vi "Module - Page Setup.vi"(11 "Stop":bool) -> ()   [LabVIEW 2020]
uses:
  Control/Setup - Sequence Data v2.ctl
  Control/Setup - Single Sequence.ctl
  Control/Setup - State.ctl
  Control/Data to Execute.ctl
  Control/Transaction Info.ctl
  Control/Product Info.ctl
  Control/Acceptance Criteria Info.ctl
  Control/Execution Info.ctl
  Control/Results Info.ctl
  Control/State - FGV.ctl
  Control/State - eFGV.ctl
  Control/Section.ctl
  <vilib>/Utility/NIReport.llb/Report Type.ctl
  7311f70c-db24-4098-937e-a840d3f1464f.vi
  babc2730-5d00-47f3-8067-32ba08f41054.vi
  3b850bdc-189a-44ac-97c7-3d94fde3370d.vi
  472a6105-114d-4794-aef6-48c339f41fe4.vi
  b5994df8-9a62-4c2b-b0b7-1cda760cb50f.vi
  133289ce-597c-4077-9071-527faaeab83e.vi
  50162af0-f45e-4f35-a68f-88f28c3fa732.vi
  <vilib>/Utility/config.llb/Read Key (String).vi
  <vilib>/addons/_office/excel.llb/Excel Get Data ([str]).vi
  <vilib>/Comparison/Equal/Equal Functor/Equal Functor.lvclass
  <vilib>/Comparison/Less/Less Functor/Less Functor.lvclass
  <vilib>/Utility/NIReport.llb/NI_report.lvclass
  <vilib>/Utility/config.llb/NI_LVConfig.lvlib
  <vilib>/Utility/file.llb/Read Delimited Spreadsheet (string).vi
  <vilib>/Utility/NIReport.llb/NI_ReportGenerationCore.lvlib
  <vilib>/Utility/NIReport.llb/Excel/NI_Excel.lvclass
  <vilib>/addons/_office/NI_ReportGenerationToolkit.lvlib
panel:
  out "Label.Test System":string="Test System"
  out "Label.Working Pressure":string="Working Pressure"
  out "Label.Test Doc No":string="Test Doc. No./Ref."
  out "Label.Product Category":string="Product Category "
  out "Label.NCR No":string="NCR No."
  out "Label.Operation No":string="Operation No.*"
  out "Label.Material":string="Material*"
  out "Label.Customer":string="Customer"
  out "Label.Project":string="Project*"
  out "Label.RefOrderNo":string="Ref. Order No.*"
  out "Label.OrderNumber":string="Order Number*"
  out "Run No.":string="99"
  in  "Label.Sensor 3":string="Sensor" caption="Sensor"
  in  "Add Additional Ref Procedure":bool caption="Add Sensor"
  in  "Remove Additional Ref Procedure":bool caption="Remove Sensor"
  in  "Table.Procedure No./Ref.":i32(listbox)
  in  "Listbox.PSL":string(combo) caption="PSL"
  in  "Listbox.Rev.":string(combo) caption="Rev."
  in  "Listbox.Additional Procedures No./Ref.":string(combo) caption="Additional Procedures No./Ref."
  in  "Label.Production Order Details":string="Production Order Details" caption="Production Order Details"
  out "Indicator.Sub Operation":string caption="Sub Operation"
  out "Indicator.Confirmation No":u32 caption="Confirmation No"
  out "Indicator.Operation":string caption="Operation"
  out "Indicator.Sequence No":u16 caption="Sequence No"
  out "Indicator.Order Number":u32 caption="Order Number"
  in  "Desc.TestSystem":string="SUT1"
  in  "Desc.ProductCategory":string="Single Unit Test"
  out "1D Results":string[](array[string])
  in  "Label.Sensor 2":string="Sensor" caption="Sensor"
  in  "Enum.Pressure stabilize wait time":enum16{"seconds", "minutes"}(ring)
  in  "Pressure stabilize wait time":dbl=30.0 caption="Test Pressure Drop Rate every" min=0.0 max=100.0
  in  "Enum.Permitted Hold Pressure Drop":enum16{"%", "psi"}(ring)
  in  "Enum.Max Start Hold Pressure":enum16{"%", "psi"}(ring)
  in  "Permitted Hold Pressure Drop":dbl=3.0 caption="Permitted Holding Pressure Drop" min=0.0 max=100.0
  in  "Max Start Hold Pressure":dbl=3.0 caption="Maximum Start of Holding Pressure" min=0.0 max=100.0
  in  "Sales Order":string
  in  "Item No.":string
  in  "Customer":string
  in  "NCR No. 2":string caption="Operation No.*"
  in  "Load Excel":bool
  in  "template (empty)":path
  in  "Tab Control":enum32{"Test", "Misc."}(tab)
  in  "ComboBox.SelectTestSequence":string(combo) caption="Test Sequence"
  in  "Remove Multi test":bool caption="Remove Sensor"
  in  "Add Multi test":bool caption="Add Sensor"
  out "Setup-Sequence Data":T1={"Seq.Done"="\nSts.", "Label.RunSeq"="\nRun", "Label.TestSeq"="Test Seq.", "Label.SeqNo"="\nNo.", "Seq.No 5"="\nTest Requirement", "Seq.No 6"="\nVariance", "Seq.No 7"="Test\nProcedure", "Seq.No 8"="\nSect.", "Seq.No 9"="Test\nSystem", "Seq.No 10"="\nTest Media", "Seq.No 11"="Test Pressure ", "Seq.No 12"="\nCycle", "Seq.No 13"="Hold. time\n(hh:mm)", "Seq.No 14"="\nChart Scale", "Seq.No 15"="\nBD", "Seq.No 16"="Actuator\nPressure", "Seq.No 17"="Max. BD\nPressure", "Label.SelectSeq"="\nSel.", "Bool.SelectSeq"=TRUE, "Bool.RunSeq"=FALSE, "Bool.TestSeq"=TRUE, "Bool.SeqNo"=FALSE, "Label.TestGroup"="Test Grp.", "Bool.TestGroup"=FALSE, "Seq.MSHP"="MSHP\n(%)", "Seq.PHPD"="PHPD\n(%)", "Array"=[{"Seq.Select"=TRUE, "Seq.Status"=16777215, "Seq.Run"=FALSE, "Seq.TestSequence"="", "Seq.No"="", "Seq.TestReq"="", "Seq.TestProcedure"="", "Seq.Section"="", "Seq.TestPressure"="88,888", "Seq.TestGroup"="", "Seq.MSHP"=0.0, "Seq.PHPD"=0.0, "Seq.HoldingTime"="", "Seq.ChartScale"="", "Seq.ActuatorPressure"="", "Seq.MaxBDPressure"="", "Seq.BDIndicator"=FALSE, "Seq.TestMedia"="", "Seq.Variance"="AMV", "Seq.TestCycle"="", "Seq.TestSystem"=""}, {"Seq.Select"=TRUE, "Seq.Status"=16777215, "Seq.Run"=FALSE, "Seq.TestSequence"="", "Seq.No"="", "Seq.TestReq"="", "Seq.TestProcedure"="", "Seq.Section"="", "Seq.TestPressure"="", "Seq.TestGroup"="", "Seq.MSHP"=0.0, "Seq.PHPD"=0.0, "Seq.HoldingTime"="", "Seq.ChartScale"="", "Seq.ActuatorPressure"="", "Seq.MaxBDPressure"="", "Seq.BDIndicator"=FALSE, "Seq.TestMedia"="", "Seq.Variance"="AAV", "Seq.TestCycle"="", "Seq.TestSystem"=""}, {"Seq.Select"=TRUE, "Seq.Status"=16777215, "Seq.Run"=FALSE, "Seq.TestSequence"="", "Seq.No"="", "Seq.TestReq"="", "Seq.TestProcedure"="", "Seq.Section"="", "Seq.TestPressure"="", "Seq.TestGroup"="", "Seq.MSHP"=0.0, "Seq.PHPD"=0.0, "Seq.HoldingTime"="", "Seq.ChartScale"="", "Seq.ActuatorPressure"="", "Seq.MaxBDPressure"="", "Seq.BDIndicator"=FALSE, "Seq.TestMedia"="", "Seq.Variance"="PMV", "Seq.TestCycle"="", "Seq.TestSystem"=""}, {"Seq.Select"=FALSE, "Seq.Status"=16777215, "Seq.Run"=FALSE, "Seq.TestSequence"="", "Seq.No"="", "Seq.TestReq"="", "Seq.TestProcedure"="", "Seq.Section"="", "Seq.TestPressure"="", "Seq.TestGroup"="", "Seq.MSHP"=0.0, "Seq.PHPD"=0.0, "Seq.HoldingTime"="", "Seq.ChartScale"="", "Seq.ActuatorPressure"="", "Seq.MaxBDPressure"="", "Seq.BDIndicator"=FALSE, "Seq.TestMedia"="", "Seq.Variance"="", "Seq.TestCycle"="", "Seq.TestSystem"=""}, {"Seq.Select"=TRUE, "Seq.Status"=16777215, "Seq.Run"=FALSE, "Seq.TestSequence"="", "Seq.No"="", "Seq.TestReq"="", "Seq.TestProcedure"="", "Seq.Section"="", "Seq.TestPressure"="", "Seq.TestGroup"="", "Seq.MSHP"=0.0, "Seq.PHPD"=0.0, "Seq.HoldingTime"="", "Seq.ChartScale"="", "Seq.ActuatorPressure"="", "Seq.MaxBDPressure"="", "Seq.BDIndicator"=FALSE, "Seq.TestMedia"="", "Seq.Variance"="", "Seq.TestCycle"="", "Seq.TestSystem"=""}, {"Seq.Select"=FALSE, "Seq.Status"=16777215, "Seq.Run"=FALSE, "Seq.TestSequence"="", "Seq.No"="", "Seq.TestReq"="", "Seq.TestProcedure"="", "Seq.Section"="", "Seq.TestPressure"="", "Seq.TestGroup"="", "Seq.MSHP"=0.0, "Seq.PHPD"=0.0, "Seq.HoldingTime"="", "Seq.ChartScale"="", "Seq.ActuatorPressure"="", "Seq.MaxBDPressure"="", "Seq.BDIndicator"=FALSE, "Seq.TestMedia"="", "Seq.Variance"="", "Seq.TestCycle"="", "Seq.TestSystem"=""}, {"Seq.Select"=FALSE, "Seq.Status"=16777215, "Seq.Run"=FALSE, "Seq.TestSequence"="", "Seq.No"="", "Seq.TestReq"="", "Seq.TestProcedure"="", "Seq.Section"="", "Seq.TestPressure"="", "Seq.TestGroup"="", "Seq.MSHP"=0.0, "Seq.PHPD"=0.0, "Seq.HoldingTime"="", "Seq.ChartScale"="", "Seq.ActuatorPressure"="", "Seq.MaxBDPressure"="", "Seq.BDIndicator"=FALSE, "Seq.TestMedia"="", "Seq.Variance"="", "Seq.TestCycle"="", "Seq.TestSystem"=""}, {"Seq.Select"=FALSE, "Seq.Status"=16777215, "Seq.Run"=FALSE, "Seq.TestSequence"="", "Seq.No"="", "Seq.TestReq"="", "Seq.TestProcedure"="", "Seq.Section"="", "Seq.TestPressure"="", "Seq.TestGroup"="", "Seq.MSHP"=0.0, "Seq.PHPD"=0.0, "Seq.HoldingTime"="", "Seq.ChartScale"="", "Seq.ActuatorPressure"="", "Seq.MaxBDPressure"="", "Seq.BDIndicator"=FALSE, "Seq.TestMedia"="", "Seq.Variance"="", "Seq.TestCycle"="", "Seq.TestSystem"=""}, {"Seq.Select"=FALSE, "Seq.Status"=16777215, "Seq.Run"=FALSE, "Seq.TestSequence"="", "Seq.No"="", "Seq.TestReq"="", "Seq.TestProcedure"="", "Seq.Section"="", "Seq.TestPressure"="", "Seq.TestGroup"="", "Seq.MSHP"=0.0, "Seq.PHPD"=0.0, "Seq.HoldingTime"="", "Seq.ChartScale"="", "Seq.ActuatorPressure"="", "Seq.MaxBDPressure"="", "Seq.BDIndicator"=FALSE, "Seq.TestMedia"="", "Seq.Variance"="", "Seq.TestCycle"="", "Seq.TestSystem"=""}, {"Seq.Select"=FALSE, "Seq.Status"=16777215, "Seq.Run"=FALSE, "Seq.TestSequence"="", "Seq.No"="", "Seq.TestReq"="", "Seq.TestProcedure"="", "Seq.Section"="", "Seq.TestPressure"="", "Seq.TestGroup"="", "Seq.MSHP"=0.0, "Seq.PHPD"=0.0, "Seq.HoldingTime"="", "Seq.ChartScale"="", "Seq.ActuatorPressure"="", "Seq.MaxBDPressure"="", "Seq.BDIndicator"=FALSE, "Seq.TestMedia"="", "Seq.Variance"="", "Seq.TestCycle"="", "Seq.TestSystem"=""}]}
  out "Label.AutoStop":string="Automatic Stop Test After the 'Stop' Marker"
  out "Header multi-test 3":T3={"EqnHeader.TypeID"="Type ID", "EqnHeader.TypeDesc"="\nType Description", "EqnHeader.ID"="\nEquipment ID", "EqnHeader.Description"="\nEquipment Description", "EqnHeader.SerialNo"="\nSerial No.", "EqnHeader.NextCalDate"="\nNext Cal. Date", "EqnHeader.LP"="\nLP"}
  in  "Remove Sensor":bool
  in  "Add Sensor":bool
  in  "Label.Sensor":string="Equipments" caption="Sensor"
  in  "Table.Sensor":i32(listbox)=1 caption="Detail Sensor"
  out "Output Set Description":string caption="Output Set Company"
  in  "ListBox.Output Set":string(combo)="1001" caption="Output Set"
  in  "Label.Result":string="Results" caption="Result"
  in  "List.Sensor":string(combo)="ASDFGGG"
  in  "Label.Execution":string="Execution" caption="Execution"
  out "Auto Stop Test":bool caption="Automatic Stop Test after Hold Time Countdown"
  in  "Auto Set Marker":bool=TRUE caption="Automatic Set 'Start' Marker upon Pressure Stabilized"
  in  "Pressure Unit":string="psi"
  in  "List SN":i32(listbox)
  in  "Test System Description":string
  in  "Rework":bool
  in  "Ref Order No.":string caption="Ref. Order No.*"
  in  "NCR No.":string
  in  "Procedure No./Ref.":string(combo)="X-355536-01-01" caption="Test Doc. No./Ref."
  in  "Save Transaction":bool
  in  "Edit Transaction":bool
  in  "Tab Control 2":T4(tab)
  in  "NewTransaction":bool
  in  "Copy Transaction":bool
  in  "Remove SN":bool
  in  "Add SN":bool
  in  "Auto":bool
  in  "Notes":string
  in  "Input SN":string
  in  "Working Pressure":string="10,000"
  in  "Test Category":string
  in  "Test System":string(combo)="SUT1"
  in  "PSL":string="3"
  in  "Rev.":string="02"
  in  "Product Category":string(combo)="SUT"
  in  "BOM Rev.":string
  in  "Material Description":string
  in  "Material":string caption="Material*"
  in  "Project":string caption="Project*"
  in  "Customer Description":string caption="Customer"
  in  "Quantity":u16=1 caption="Quantity*" min=1 step=1
  in  "Order Number":string caption="Order Number*"
  in  "Search":bool
  out "Transaction Number":string="1232154652" caption="Transaction No."
  # "SETUP"
  # "Rev.."
  # "PSL"
  # "on Top of the Test Pressure"
  # "Per Hour (vs. Start Holding Pressure)"
  # "Maximum Start of Holding Pressure"
  # "Pressure Holding Pressure Drop"
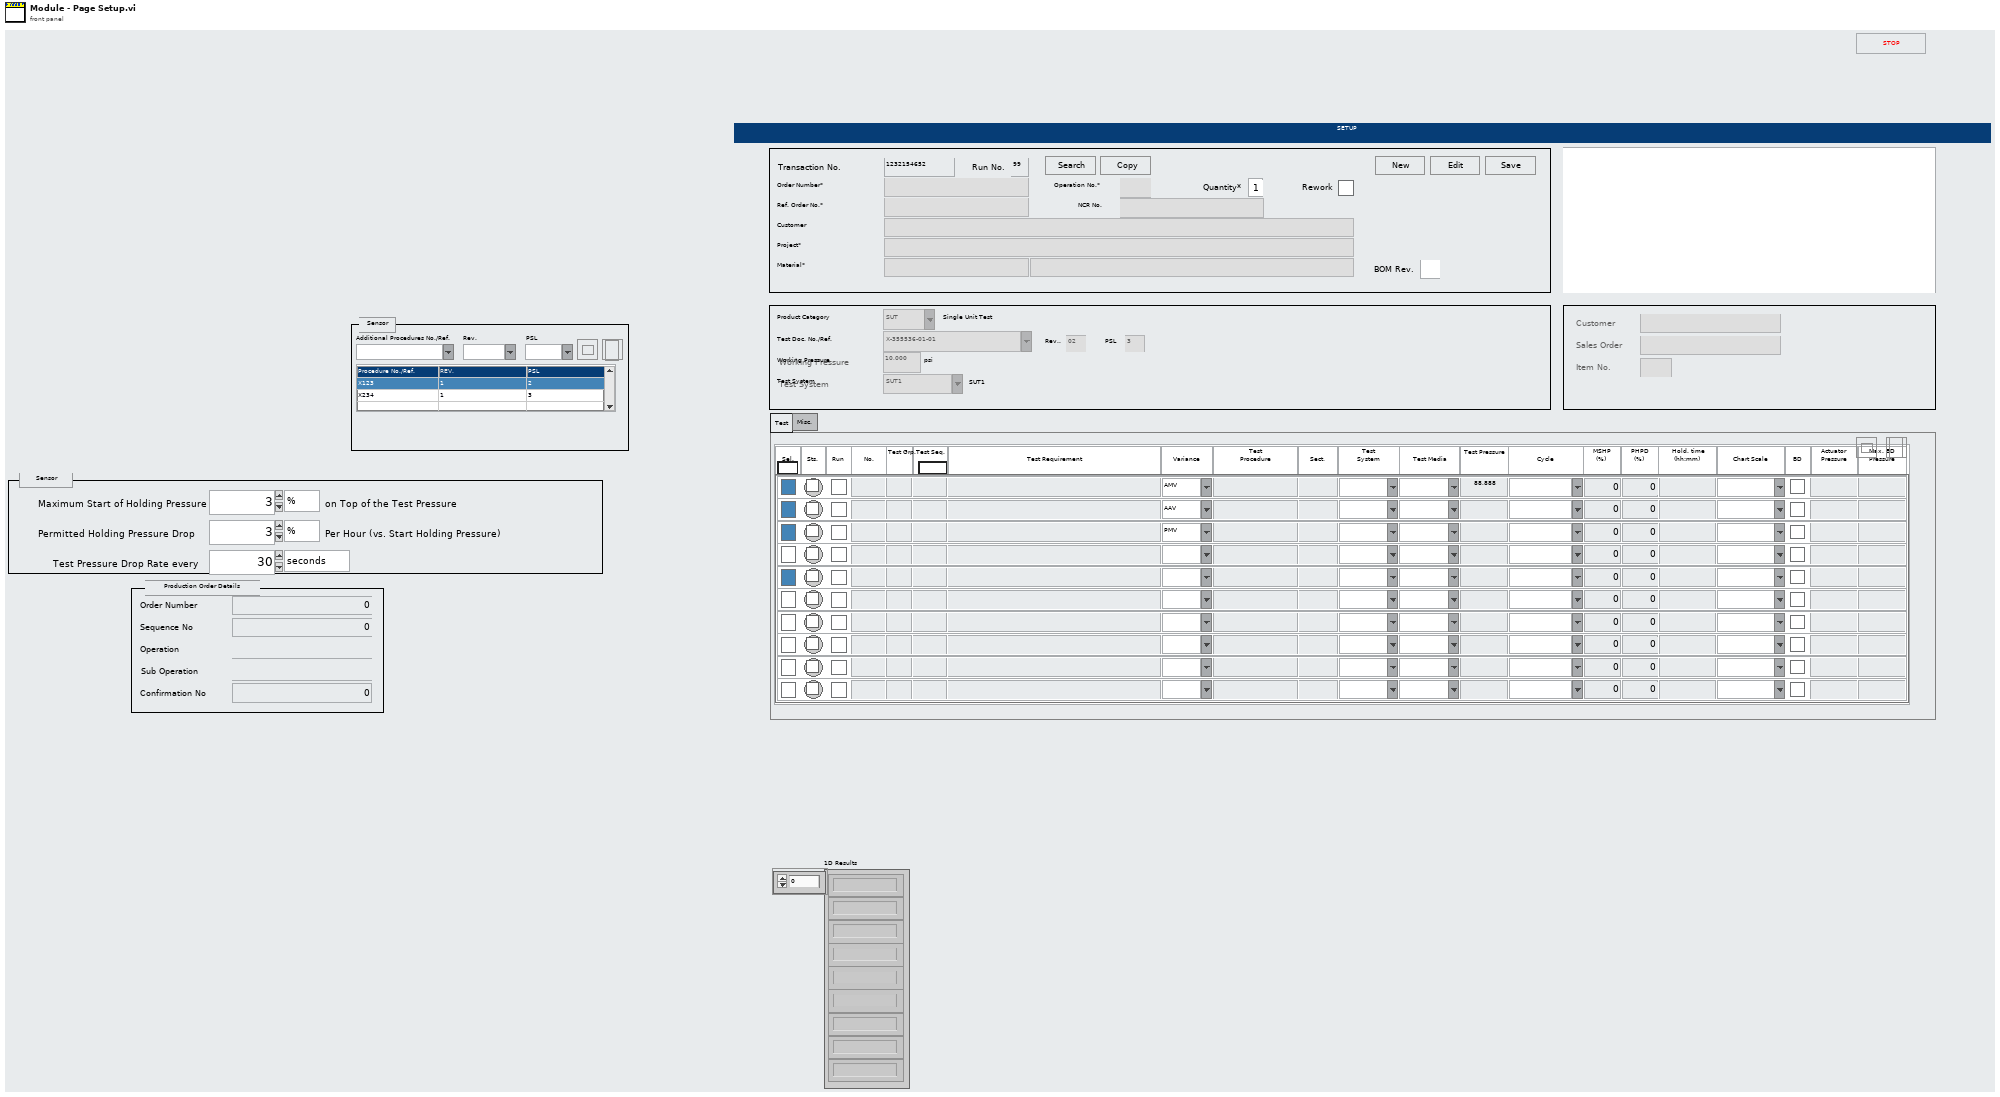
[diagram p1: front panel]
types:
  T1 = typedef "Setup - Sequence Data v2.ctl" = cluster{"Seq.Done":string, "Label.RunSeq":string, "Label.TestSeq":string, "Label.SeqNo":string, "Seq.No 5":string, "Seq.No 6":string, "Seq.No 7":string, "Seq.No 8":string, "Seq.No 9":string, "Seq.No 10":string, "Seq.No 11":string, "Seq.No 12":string, "Seq.No 13":string, "Seq.No 14":string, "Seq.No 15":string, "Seq.No 16":string, "Seq.No 17":string, "Label.SelectSeq":string, "Bool.SelectSeq":bool, "Bool.RunSeq":bool, "Bool.TestSeq":bool, "Bool.SeqNo":bool, "Label.TestGroup":string, "Bool.TestGroup":bool, "Seq.MSHP":string, "Seq.PHPD":string, "Array":T2[]}
  T2 = typedef "Setup - Single Sequence.ctl" = cluster{"Seq.Select":bool, "Seq.Status":u32, "Seq.Run":bool, "Seq.TestSequence":string, "Seq.No":string, "Seq.TestReq":string, "Seq.TestProcedure":string, "Seq.Section":string, "Seq.TestPressure":string, "Seq.TestGroup":string, "Seq.MSHP":dbl, "Seq.PHPD":dbl, "Seq.HoldingTime":string, "Seq.ChartScale":string, "Seq.ActuatorPressure":string, "Seq.MaxBDPressure":string, "Seq.BDIndicator":bool, "Seq.TestMedia":string, "Seq.Variance":string, "Seq.TestCycle":string, "Seq.TestSystem":string}
  T3 = cluster{"EqnHeader.TypeID":string, "EqnHeader.TypeDesc":string, "EqnHeader.ID":string, "EqnHeader.Description":string, "EqnHeader.SerialNo":string, "EqnHeader.NextCalDate":string, "EqnHeader.LP":string}
  T4 = enum32{"Others                ", "Multi-tests       "}
  T5 = typedef "Data to Execute.ctl" = cluster{"Transaction Info":T6, "Product Info":T7, "Misc - Additional Refs":string[][], "Misc - Sensors":string[][], "Misc - Tools":string[][], "Acceptance Criteria Info":T8, "Execution Info":T9, "Results Info":T10, "Notes":string}
  T6 = typedef "Transaction Info.ctl" = cluster{"Transaction Number":string, "Order Number":string, "Quantity":u16, "Customer":string, "Customer Description":string, "Project":string, "Sales Order":string, "Material":string, "Material Description":string, "Rework":bool, "NCR No.":string, "Ref Order No.":string, "Item No.":string, "BOM Rev.":string}
  T7 = typedef "Product Info.ctl" = cluster{"Product Category":string, "Procedure No./Ref.":string, "Test System":string, "Test System Description":string, "Working Pressure":string, "Pressure Unit":string, "Rev.":string, "PSL":string}
  T8 = typedef "Acceptance Criteria Info.ctl" = cluster{"Max Start Hold Pressure":dbl, "Enum.Max Start Hold Pressure":enum16{"%", "psi"}, "Permitted Hold Pressure Drop":dbl, "Enum.Permitted Hold Pressure Drop":enum16{"%", "psi"}, "Pressure stabilize wait time":dbl, "Enum.Pressure stabilize wait time":enum16{"seconds", "minutes"}}
  T9 = typedef "Execution Info.ctl" = cluster{"Auto Set Marker":bool, "Auto Stop Test":bool}
  T10 = typedef "Results Info.ctl" = cluster{"ListBox.Output Set":string, "Output Set Description":string}
  T11 = cluster{"T_Out":i32, "Event Ref":refnum<event-registration>, "Product Category":string, "Seq.AllList":cluster{"Seq.Select":bool, "Seq.Status":u32, "Seq.Run":bool, "Seq.TestSequence":string, "Seq.No":string, "Seq.ReqID":string, "Seq.TestReq":string, "Seq.Variance":string, "Seq.TestProcedure":string, "Seq.Section":string, "Seq.TestBunker":string, "Seq.TestMedia":string, "Seq.TestPressure":string, "Seq.Cycle":string, "Seq.HoldingTime":string, "Seq.ChartScale":string, "Seq.BDIndicator":string, "Seq.ActuatorPressure":string, "Seq.MaxBDPressure":string}[], "Seq.ShownList":cluster{"Seq.Select":bool, "Seq.Status":u32, "Seq.Run":bool, "Seq.TestSequence":string, "Seq.No":string, "Seq.ReqID":string, "Seq.TestReq":string, "Seq.Variance":string, "Seq.TestProcedure":string, "Seq.Section":string, "Seq.TestBunker":string, "Seq.TestMedia":string, "Seq.TestPressure":string, "Seq.Cycle":string, "Seq.HoldingTime":string, "Seq.ChartScale":string, "Seq.BDIndicator":string, "Seq.ActuatorPressure":string, "Seq.MaxBDPressure":string}[], "Seq.HiddenList":cluster{"Seq.Select":bool, "Seq.Status":u32, "Seq.Run":bool, "Seq.TestSequence":string, "Seq.No":string, "Seq.ReqID":string, "Seq.TestReq":string, "Seq.Variance":string, "Seq.TestProcedure":string, "Seq.Section":string, "Seq.TestBunker":string, "Seq.TestMedia":string, "Seq.TestPressure":string, "Seq.Cycle":string, "Seq.HoldingTime":string, "Seq.ChartScale":string, "Seq.BDIndicator":string, "Seq.ActuatorPressure":string, "Seq.MaxBDPressure":string}[], "Procedure No.":string, "File String":string[], "Data to Execute":T5, "Bool Tracker":cluster{"Bool.SelectSeq":bool, "Bool.RunSeq":bool, "Bool.TestSeq":bool, "Bool.NoSeq":bool}}
  T12 = typedef "Setup - State.ctl" = enum16{"Init", "Register Event", "Read Config File", "Get Output Set List", "Get procedure list", "Idle", "Get product info", "Read sequence csv", "Get Sequence List", "Get Transaction Info", "Get product Info", "Get Misc - Additional Refs", "Get Misc - Sensors", "Get Misc - Tools", "Get Misc - Accept Criteria", "Get Misc - Execution", "Get Misc - Results", "Get Misc - Notes", "Check Folder Exist", "Create Folder", "Send to Execute", "Close"}
  T13 = typedef "State - FGV.ctl" = enum16{"Write", "Read"}
  T14 = typedef "State - eFGV.ctl" = enum16{"Init", "Read", "Write", "Exit"}
  T15 = typedef "Section.ctl" = enum16{"Software Setup", "Config", "Setup", "Network Stream", "MQTT Client", "Setting", "Sample Interval", "Calibration", "Pre-Ranging", "Overrun", "Static", "Filter", "Properties", "Alarm", "Device", "Logging"}
  T16 = cluster{"Seq.Select":bool, "Seq.Status":u32, "Seq.Run":bool, "Seq.TestSequence":string, "Seq.No":string, "Seq.ReqID":string, "Seq.TestReq":string, "Seq.Variance":string, "Seq.TestProcedure":string, "Seq.Section":string, "Seq.TestBunker":string, "Seq.TestMedia":string, "Seq.TestPressure":string, "Seq.Cycle":string, "Seq.HoldingTime":string, "Seq.ChartScale":string, "Seq.BDIndicator":string, "Seq.ActuatorPressure":string, "Seq.MaxBDPressure":string}[]
  T17 = enum8{"Enabled", "Disabled", "Disabled and Grayed Out"}
  T18 = enum16{"maximized", "minimized", "normal", "no change"}
  T19 = typedef "NI_ReportGenerationCore.lvlib/Report Type.ctl" = enum16{"HTML", "Word", "Excel"}
  T20 = typedef "NI_LVConfig.lvlib/Config Data RefNum.ctl" = refnum<k1>
  T21 = cluster{"Seq.TestSequence":string, "Setup - Sequence Data":T2}
  T22 = cluster{"Seq.TestSequence":string, "Setup - Sequence Data":T2}[]
  T23 = cluster{"Seq.No":string, "Setup - Sequence Data":T2}
  T24 = cluster{"Seq.No":string, "Setup - Sequence Data":T2}[]
  T25 = cluster{"Type":string, "ID":string, "Description":string, "Serial No.":string, "Low Pressure?":bool}
  T26 = cluster{"Transaction Number":string, "Order Number":string, "Quantity":u16, "Customer":string, "Customer Description":string, "Project":string, "Sales Order":string, "Material":string, "Material Description":string, "Rework":bool, "NCR No.":string, "Ref Order No.":string, "Item No.":string, "BOM Rev.":string}
  T27 = cluster{"Product Category":string, "Procedure No./Ref.":string, "Test System":string, "Test System Description":string, "Working Pressure":string, "Pressure Unit":string, "Rev.":string, "PSL":string}
  T28 = cluster{"Max Start Hold Pressure":dbl, "Enum.Max Start Hold Pressure":enum16{"%", "psi"}, "Permitted Hold Pressure Drop":dbl, "Enum.Permitted Hold Pressure Drop":enum16{"%", "psi"}, "Pressure stabilize wait time":dbl, "Enum.Pressure stabilize wait time":enum16{"seconds", "minutes"}}
  T29 = cluster{"Auto Set Marker":bool, "Auto Stop Test":bool}
  T30 = cluster{"ListBox.Output Set":string, "Output Set Description":string}
  T31 = enum32{"invalid app kind", "Development System", "Run Time System", "Student Edition", "Embedded LabVIEW", "Evaluation", "Custom"}
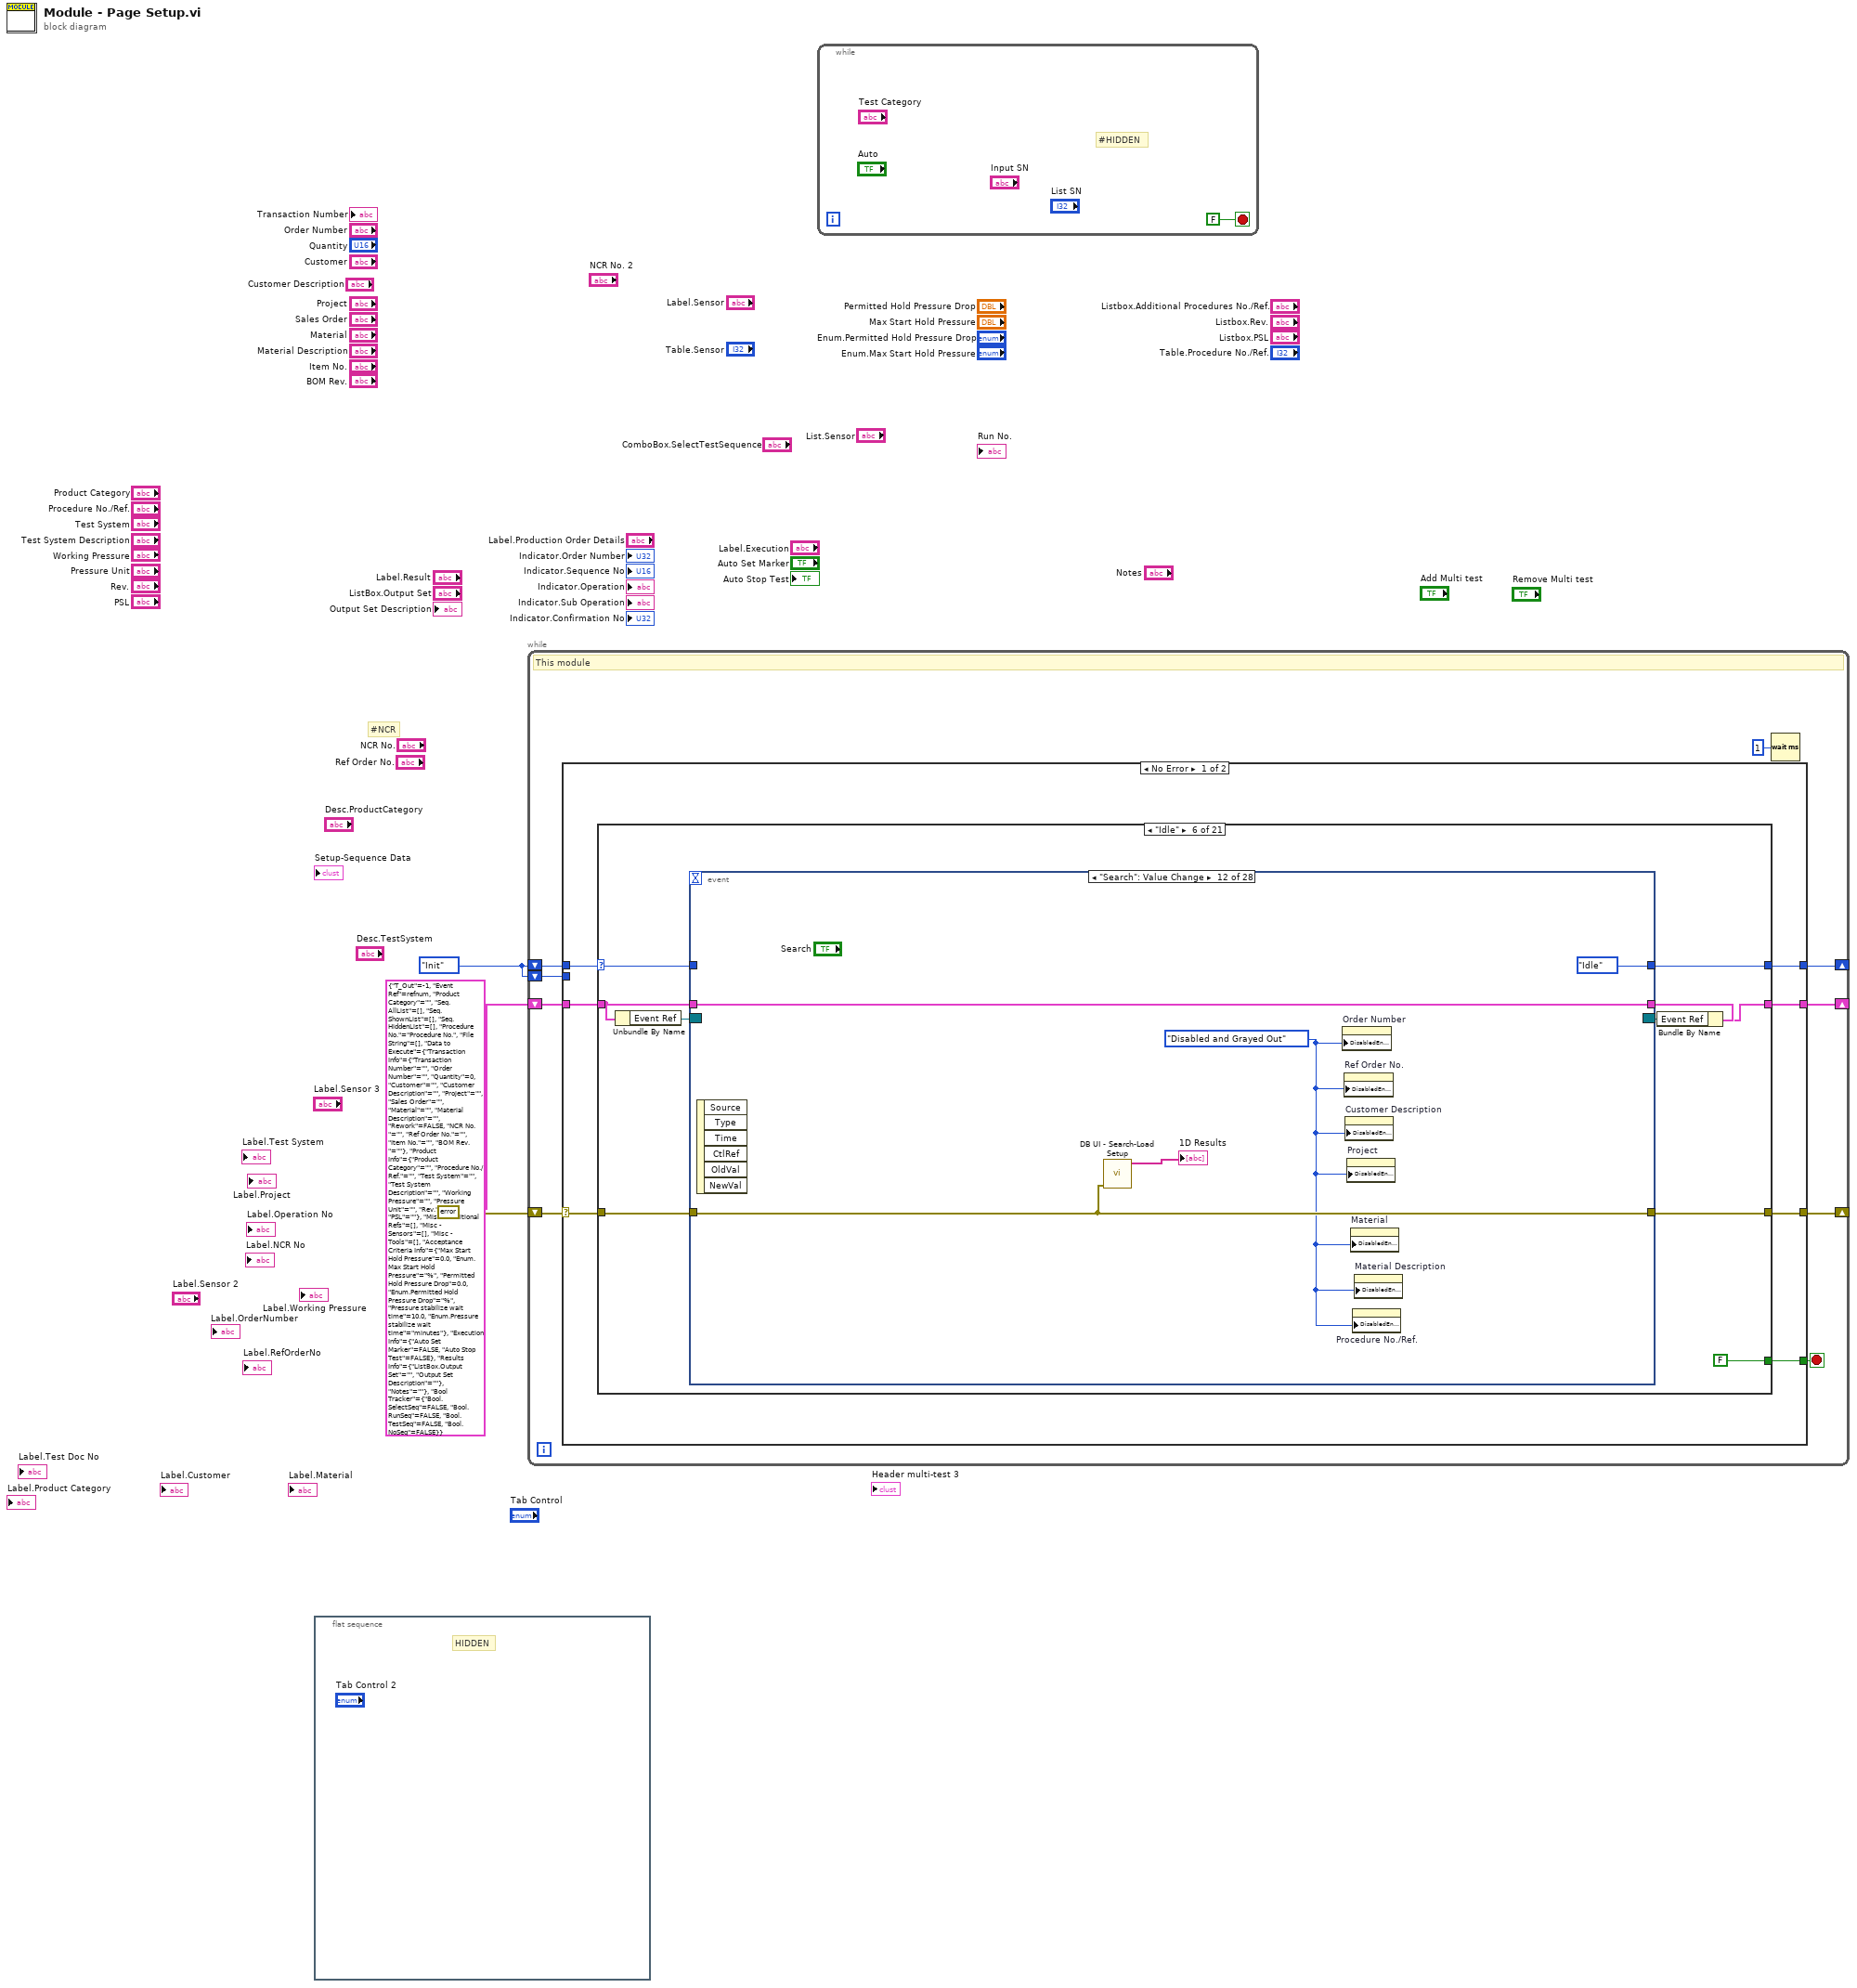
[diagram p0: block diagram]
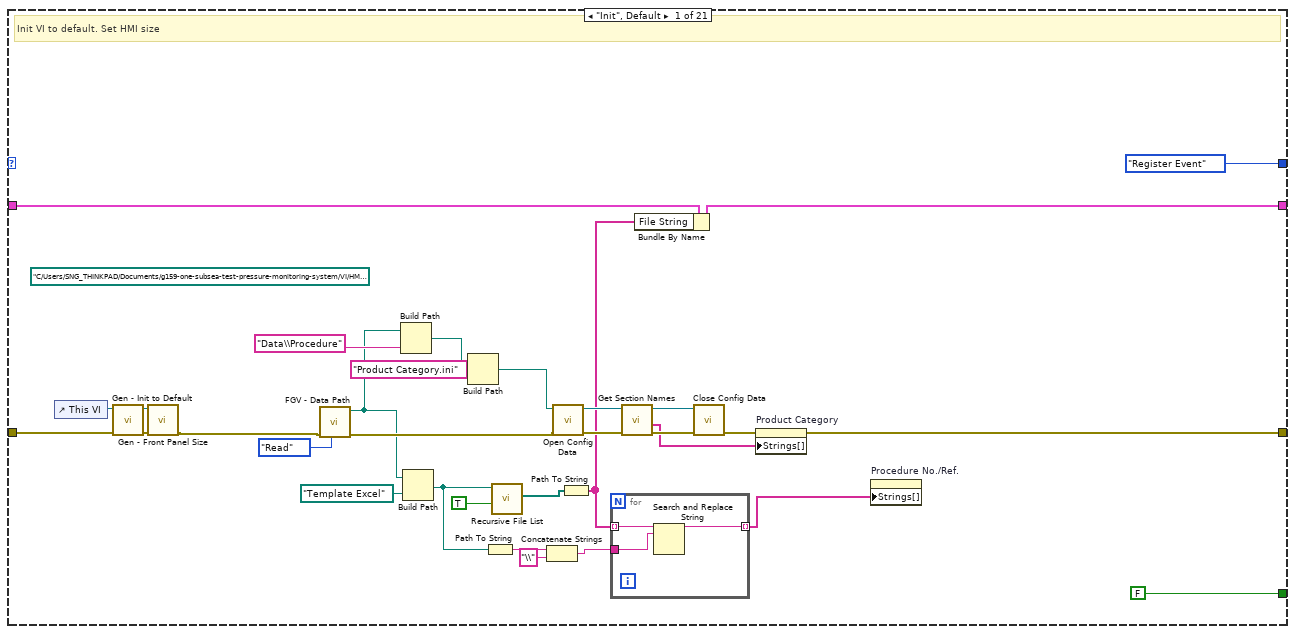
[diagram p2: hidden frame]
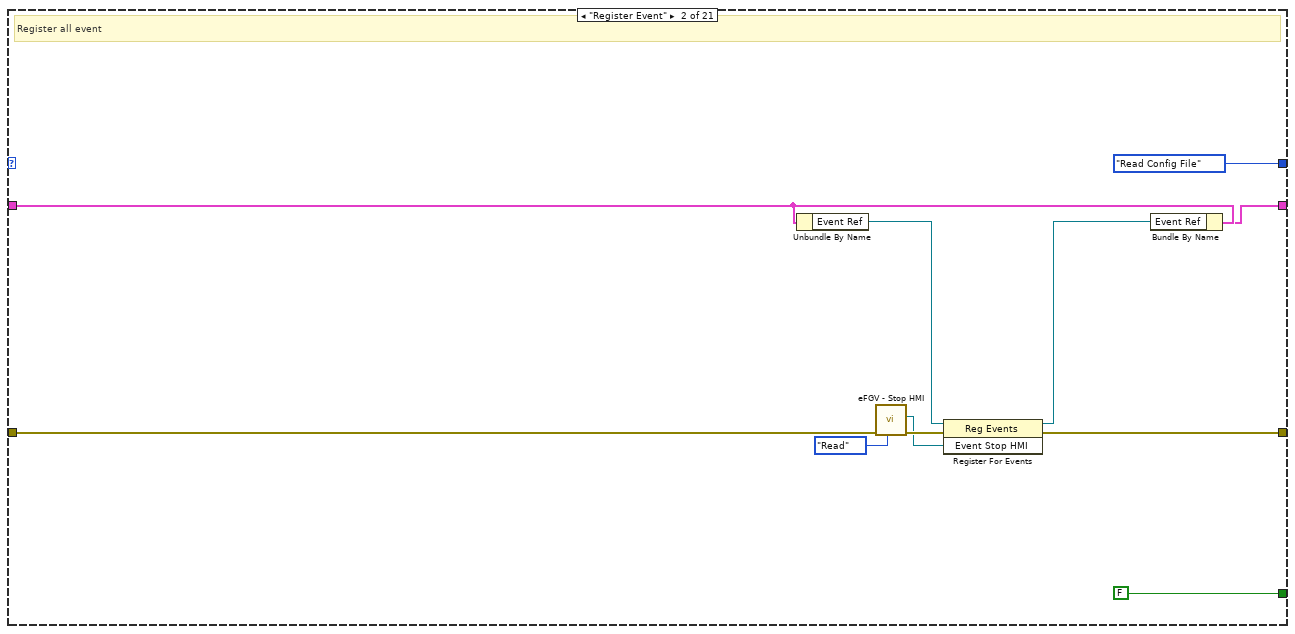
[diagram p3: hidden frame]
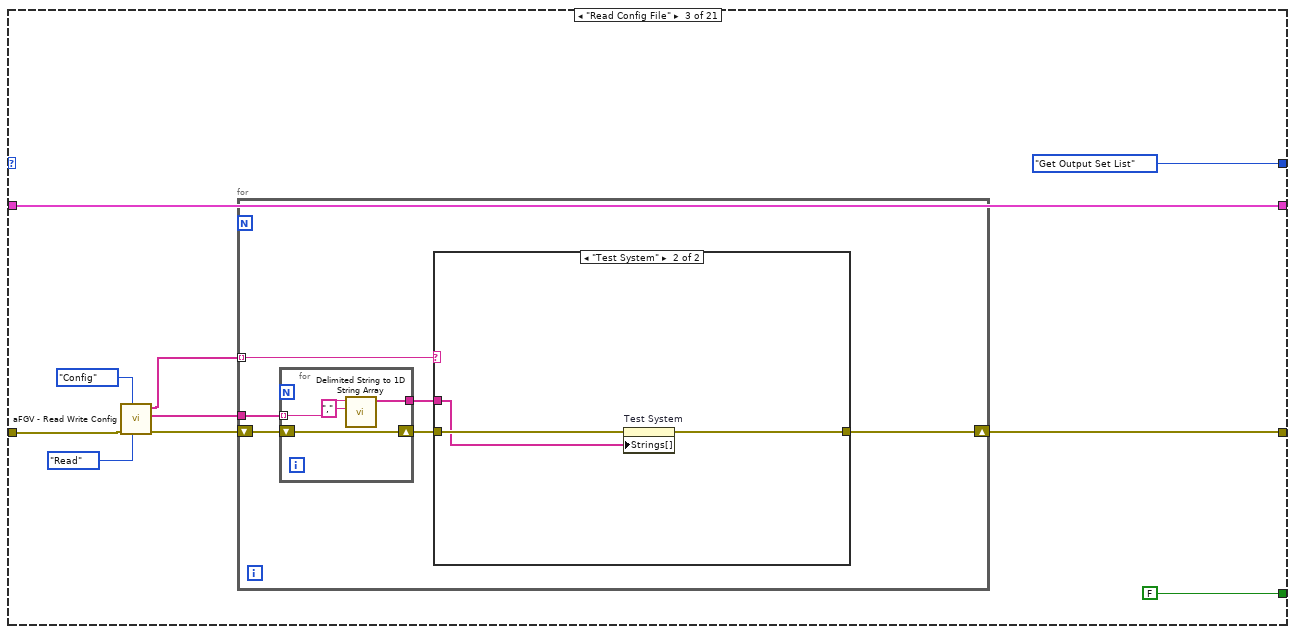
[diagram p4: hidden frame]
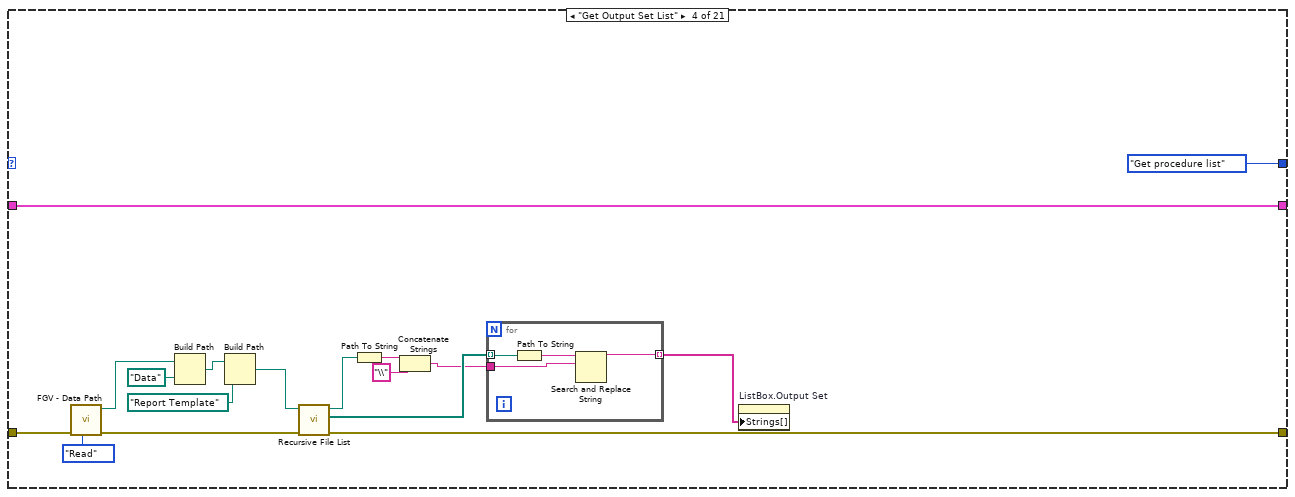
[diagram p6: hidden frame]
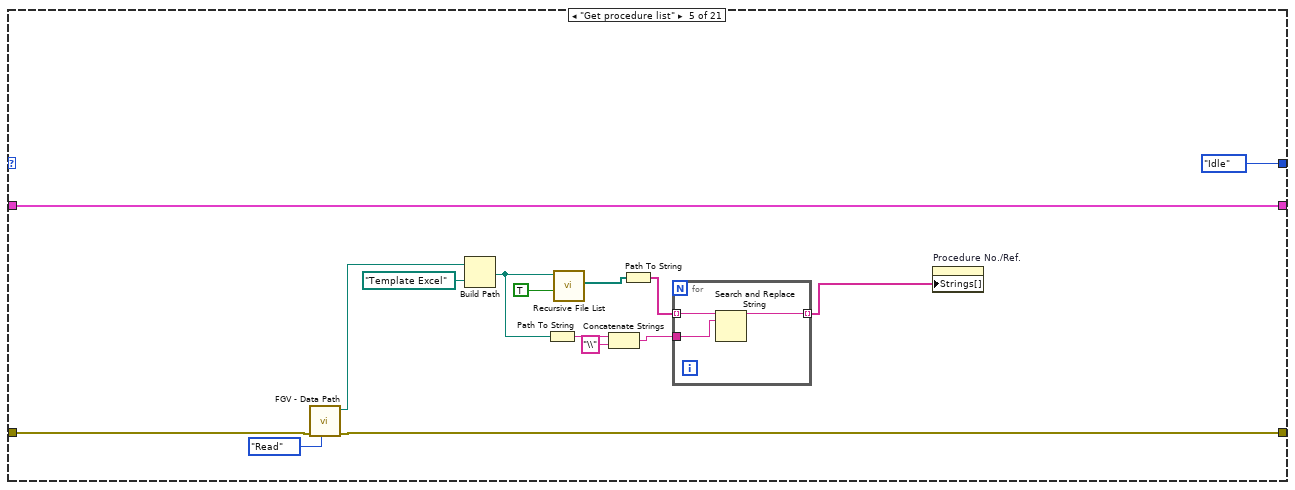
[diagram p7: hidden frame]
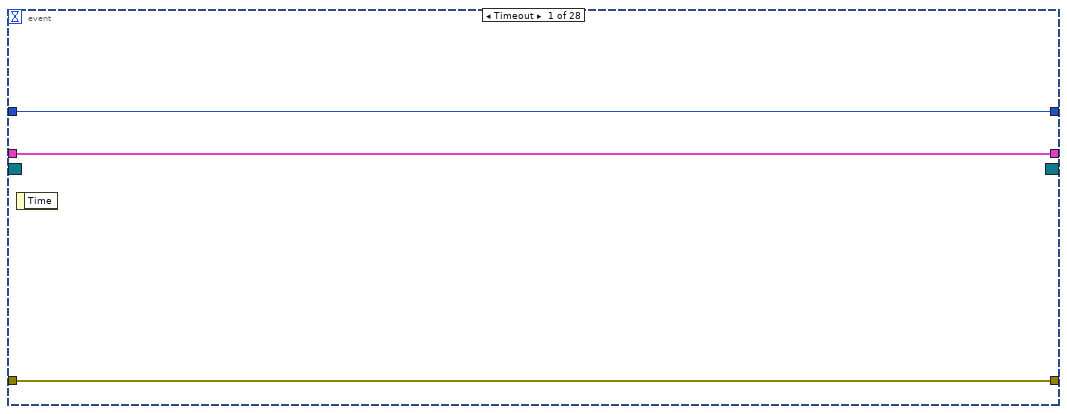
[diagram p8: hidden frame]
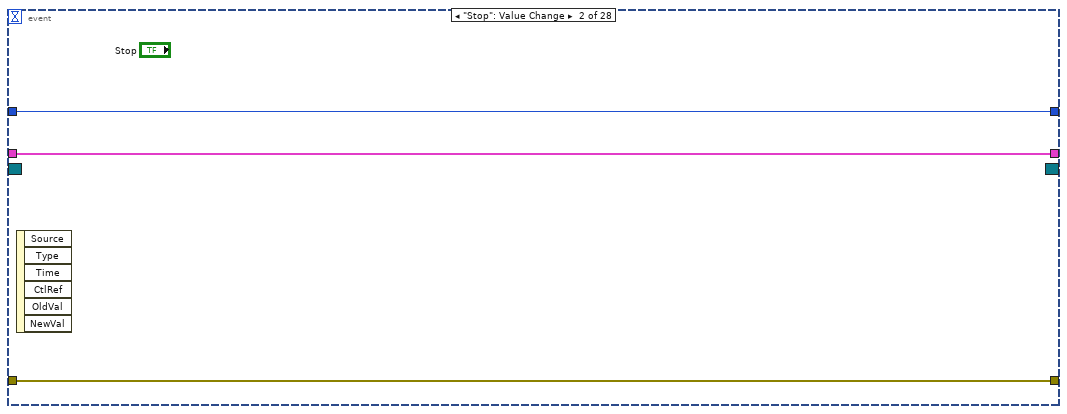
[diagram p9: hidden frame]
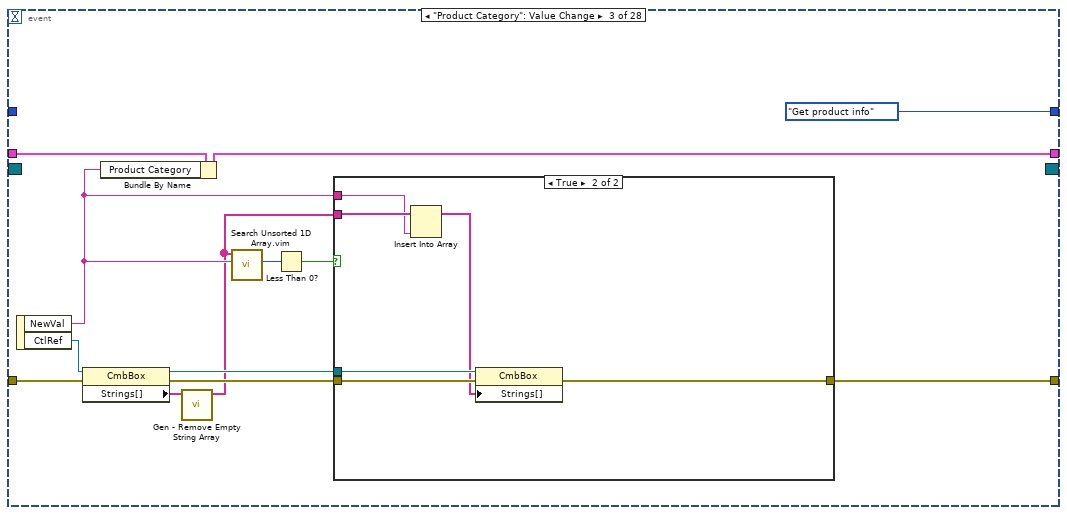
[diagram p10: hidden frame]
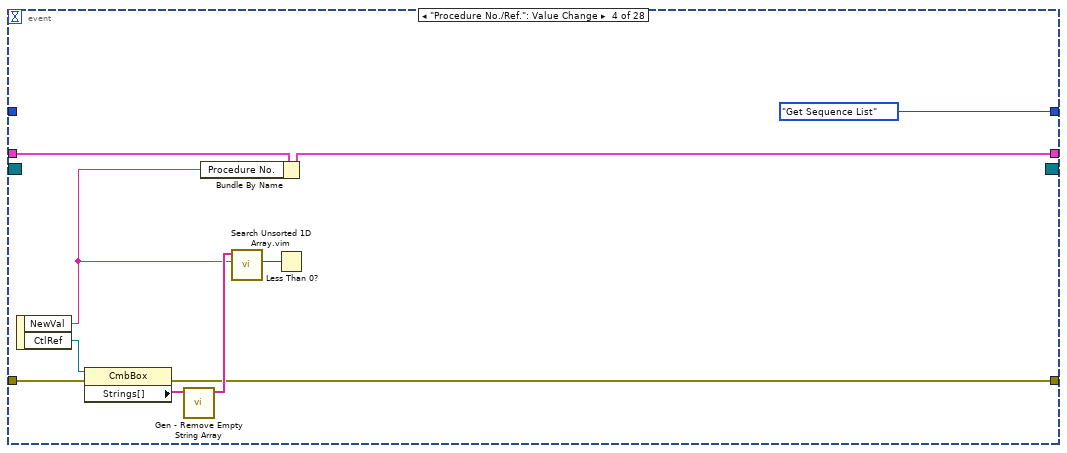
[diagram p12: hidden frame]
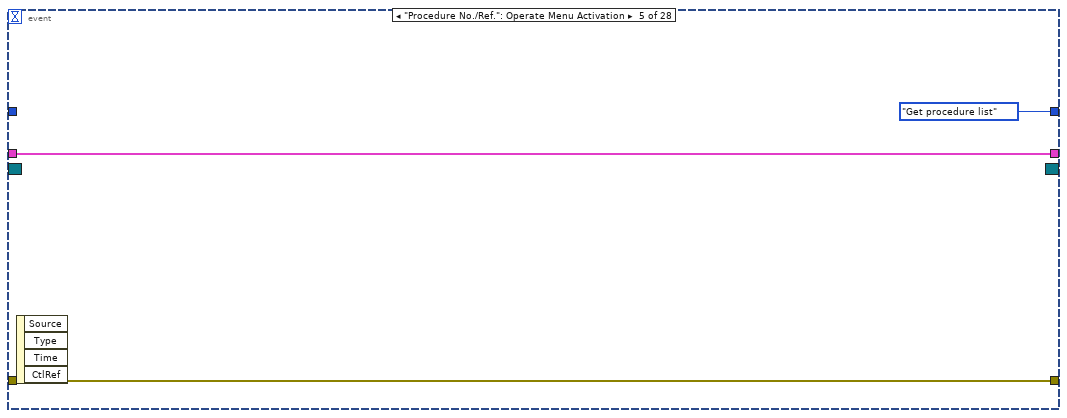
[diagram p13: hidden frame]
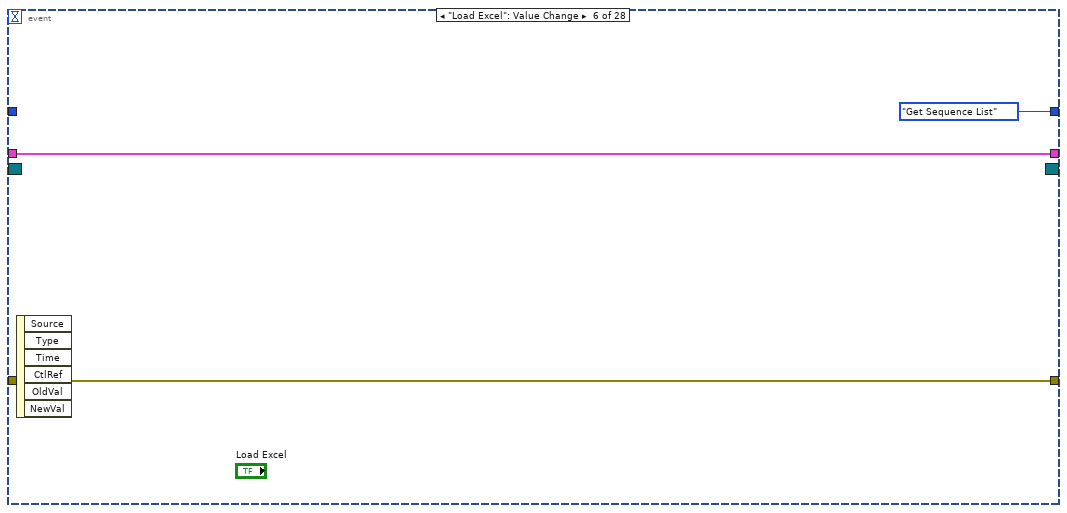
[diagram p14: hidden frame]
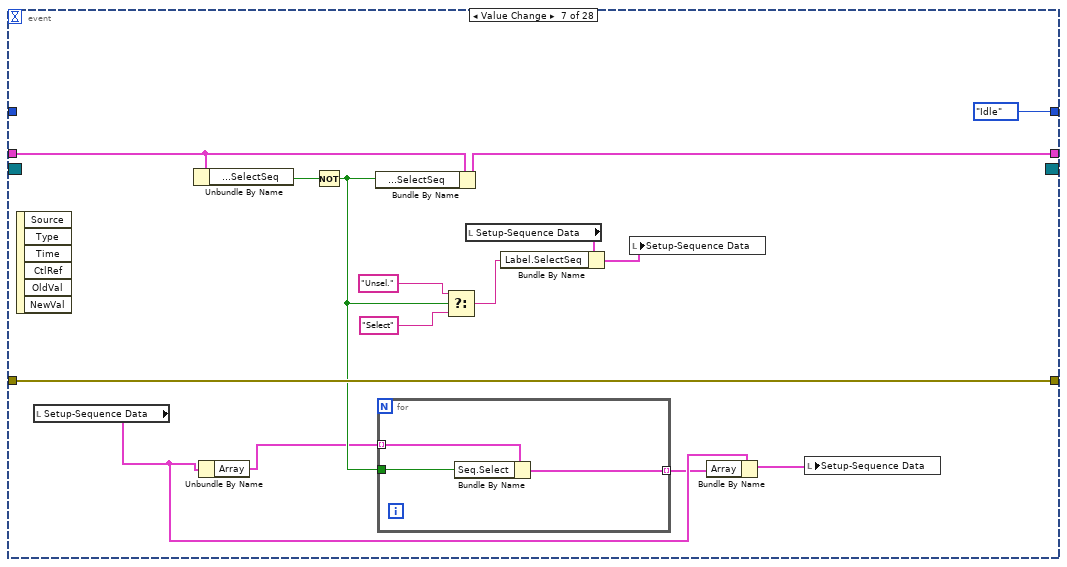
[diagram p15: hidden frame]
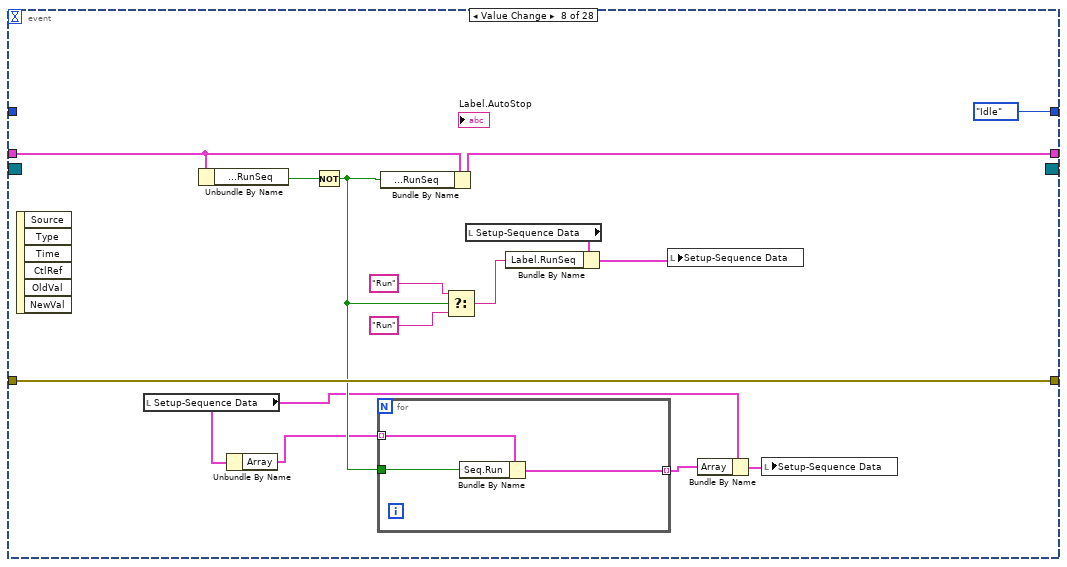
[diagram p16: hidden frame]
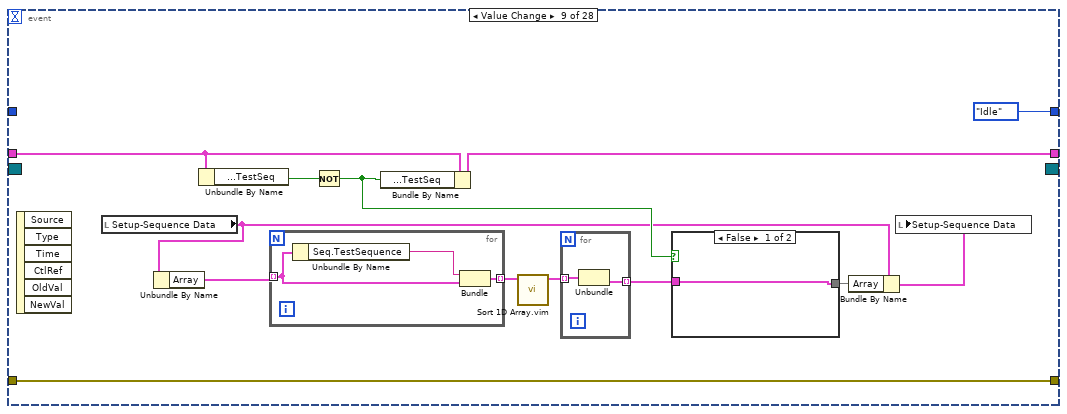
[diagram p17: hidden frame]
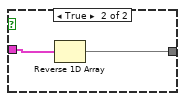
[diagram p18: hidden frame]
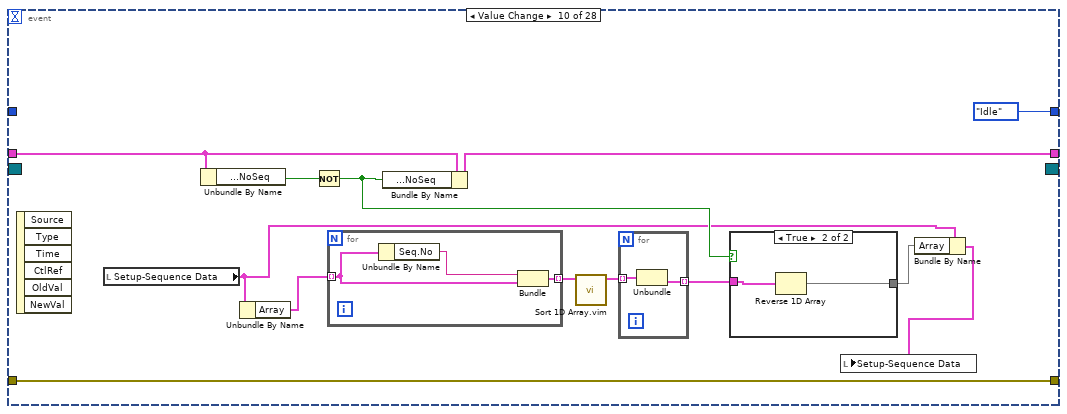
[diagram p19: hidden frame]
diagram:
  w1 = Setup_-_State."Init"
  # "#NCR"
  n1 = flat-sequence {
    frame #0 {
      # "HIDDEN"
    }
  }
  n2 = while {
    shift-right: [w8] -> _
    shift-left: w1 -> [w10]
    shift-right: [w11] -> _
    shift-left: errorcluster {"status"=FALSE, "code"=0, "source"=""} ("Error In") -> [w12]
    shift-right: [w6] -> _
    shift-left: T11 {"T_Out"=-1, "Event Ref"=refnum, "Product Category"="", "Seq.AllList"=[], "Seq.ShownList"=[], "Seq.HiddenList"=[], "Procedure No."="Procedure No.", "File String"=[], "Data to Execute"={"Transaction Info"={"Transaction Number"="", "Order Number"="", "Quantity"=0, "Customer"="", "Customer Description"="", "Project"="", "Sales Order"="", "Material"="", "Material Description"="", "Rework"=FALSE, "NCR No."="", "Ref Order No."="", "Item No."="", "BOM Rev."=""}, "Product Info"={"Product Category"="", "Procedure No./Ref."="", "Test System"="", "Test System Description"="", "Working Pressure"="", "Pressure Unit"="", "Rev."="", "PSL"=""}, "Misc - Additional Refs"=[], "Misc - Sensors"=[], "Misc - Tools"=[], "Acceptance Criteria Info"={"Max Start Hold Pressure"=0.0, "Enum.Max Start Hold Pressure"=enum."%", "Permitted Hold Pressure Drop"=0.0, "Enum.Permitted Hold Pressure Drop"=enum."%", "Pressure stabilize wait time"=10.0, "Enum.Pressure stabilize wait time"=enum."minutes"}, "Execution Info"={"Auto Set Marker"=FALSE, "Auto Stop Test"=FALSE}, "Results Info"={"ListBox.Output Set"="", "Output Set Description"=""}, "Notes"=""}, "Bool Tracker"={"Bool.SelectSeq"=FALSE, "Bool.RunSeq"=FALSE, "Bool.TestSeq"=FALSE, "Bool.NoSeq"=FALSE}} -> [w7]
    shift-left: w1 -> [w4]
    stop <- w9 stop-if-true
    # "This module"
    n3 = case shown="No Error" w12 {
      selector: w12 -> [w18 w684]
      tunnel: w10 -> [w17 w689]
      tunnel: [w19 w685] -> w11
      tunnel: [w16 FALSE] -> w9
      tunnel: [w15 w689] -> w8
      tunnel: w7 -> [w14 w688]
      tunnel: [w13 w688] -> w6
      tunnel: w4 -> [_ w681]
      frame No Error {
        n4 = case shown="\"Idle\"" w17 {
          selector: w17 -> [_ _ _ _ _ w133 _ _ _ _ _ _ _ _ _ _ _ _ _ _ w678]
          tunnel: [w39 w65 w68 w98 w113 w138 w481 w510 w536 w583 w600 w604 w610 w613 w626 w633 w640 w645 w649 w673 w679] -> w19
          tunnel: w18 -> [w51 w63 w73 w104 w114 w137 w482 w509 w537 w583 w600 w605 w611 w613 w626 w633 w640 w645 w659 w674 w680]
          tunnel: [FALSE FALSE FALSE _ _ FALSE FALSE FALSE _ FALSE _ _ _ _ _ _ _ _ _ _ TRUE] -> w16
          tunnel: [Setup_-_State."Register Event" Setup_-_State."Read Config File" Setup_-_State."Get Output Set List" Setup_-_State."Get procedure list" Setup_-_State."Idle" w135 Setup_-_State."Read sequence csv" Setup_-_State."Idle" Setup_-_State."Idle" Setup_-_State."Get product Info" Setup_-_State."Get Misc - Additional Refs" Setup_-_State."Get Misc - Sensors" Setup_-_State."Get Misc - Tools" Setup_-_State."Get Misc - Accept Criteria" Setup_-_State."Get Misc - Execution" Setup_-_State."Get Misc - Results" Setup_-_State."Get Misc - Notes" Setup_-_State."Check Folder Exist" w650 Setup_-_State."Idle" w678] -> w15
          tunnel: w14 -> [w49 w59 w75 w106 w125 w132 w480 w513 w533 w581 w599 w606 w612 w615 w625 w632 w639 w644 w656 w671 w676]
          tunnel: [w22 w57 w75 w106 w125 w130 w480 w513 w535 w579 w590 w603 w609 w615 w621 w629 w636 w643 w656 w671 w676] -> w13
          frame "Init", Default {
            (unwired) path "C:/Users/SNG_THINKPAD/Documents/g159-one-subsea-test-pressure-monitoring-system/VI/HMI/Data/Data/Procedure/Product Category.ini" ("configuration file path")
            # "Init VI to default. Set HMI size"
            n5 = control-ref of="This VI"() -> (w47:refnum<vi>)
            n6 = call "Gen - Init to Default.vi"("Error in"=w51, "This VI"=w47) -> ("Error out"=w50:errorcluster, "This VI Copy"=w46:refnum<vi>)  [unwired: 8 in]
            n7 = call "Gen - Front Panel Size.vi"("Error In"=w50, "This VI"=w46) -> ("Error Out"=w36:errorcluster)  [unwired: 9 in]
            n8 = call "FGV - Data Path.vi"("FGV State"=State_-_FGV."Read", "Error In"=w36) -> ("Error Out"=w35:errorcluster, "Path Out"=w31:path)  [unwired: 8 in]
            n9 = Build Path(base path=w31, name or relative path="Data\\Procedure") -> (appended path=w34:path)
            n10 = Build Path(base path=w31, name or relative path=path "Template Excel") -> (appended path=w27:path)
            n11 = Build Path(base path=w34, name or relative path="Product Category.ini") -> (appended path=w32:path)
            n12 = Path To String(path=w27) -> (string=w25:string)
            n13 = call <vilib>:"Recursive File List.vi"("Continue Recursing on Error? (F)"=TRUE, "Folder Path"=w27) -> ("All Files in Dir"=w28:path[])  [unwired: 5 in, 4 out]
            n14 = Concatenate Strings(w25, "\\" ("string")) -> (w23:string)
            n15 = call <vilib>:"Open Config Data.vi"("error in (no error)"=w35, "configuration file path"=w32) -> ("error out"=w45:errorcluster, "refnum"=w42:T20)  [unwired: 7 in, 1 out]
            n16 = Path To String(path=w28) -> (string=w21:string[])
            n17 = for {
              tunnel: w21 -> [w54] mode=indexing
              tunnel: w23 -> [w53]
              tunnel: [w52] -> w26 mode=indexing
              n18 = Search and Replace String(input string=w54, search string=w53) -> (result string=w52:string)  [unwired: 6 in, 3 out]
            }
            n19 = call <vilib>:"Get Section Names.vi"("error in (no error)"=w45, "refnum"=w42) -> ("error out"=w43:errorcluster, "section names"=w40:string[], "refnum out"=w44:T20)  [unwired: 7 in]
            n20 = Bundle By Name(cluster=w49, "File String"=w21) -> (w22:T11)
            n21 = call <vilib>:"Close Config Data.vi"("error in (no error)"=w43, "refnum"=w44) -> ("error out"=w41:errorcluster)  [unwired: 8 in, 1 out]
            n22 = property on="Product Category" class="CmbBox"(error in=w41, "Strings[]"=w40) -> (error out=w39:errorcluster)  [unwired: 1 in, 1 out]
            n23 = property on="Procedure No./Ref." class="CmbBox"("Strings[]"=w26) -> ()  [unwired: 2 in, 2 out]
          }
          frame "Register Event" {
            # "Register all event"
            n24 = Unbundle By Name(w59) -> ("Event Ref"=w58:refnum<event-registration>)
            n25 = call "eFGV - Stop HMI.vi"("Action"=State_-_eFGV."Read", "Error In"=w63) -> ("Error Out"=w64:errorcluster, "Event Stop HMI"=w61:refnum<user-event>)  [unwired: 7 in, 1 out]
            n26 = register-events(reference=w58, error in=w64, w61) -> (reference out=w56:refnum<event-registration>, error out=w65:errorcluster)
            n27 = Bundle By Name(cluster=w59, "Event Ref"=w56) -> (w57:T11)
          }
          frame "Read Config File" {
            n28 = call "aFGV - Read Write Config.vi"("State"=enum16{"Read", "Write", "Delete"}."Read", "Section"=Section."Config", "Error In"=w73) -> ("Error Out"=w69:errorcluster, "Data out"=w66:string[], "Key Names"=w67:string[])  [unwired: 6 in]
            n29 = for {
              shift-right: [w81] -> w68
              shift-left: w69 -> [w79]
              tunnel: w67 -> [w80] mode=indexing
              tunnel: w66 -> [w77]
              n30 = for {
                shift-right: [w85] -> w78
                shift-left: w79 -> [w85]
                tunnel: w77 -> [w84] mode=indexing
                tunnel: [w82] -> w76
                n31 = call <vilib>:"Delimited String to 1D String Array.vi"("delimiter"=",", "delimited string"=w84) -> ("string array"=w82:string[])  [unwired: 9 in]
              }
              n32 = case shown="\"Test System\"" w80 {
                tunnel: w78 -> [w86 w89]
                tunnel: [w86 w88] -> w81
                tunnel: w76 -> [_ w87]
                frame Default {
                }
                frame "Test System" {
                  n33 = property on="Test System" class="CmbBox"(error in=w89, "Strings[]"=w87) -> (error out=w88:errorcluster)  [unwired: 1 in, 1 out]
                }
              }
            }
          }
          frame "Get Output Set List" {
            n34 = call "FGV - Data Path.vi"("FGV State"=State_-_FGV."Read", "Error In"=w104) -> ("Error Out"=w99:errorcluster, "Path Out"=w103:path)  [unwired: 8 in]
            n35 = Build Path(base path=w103, name or relative path=path "Data") -> (appended path=w101:path)
            n36 = Build Path(base path=w101, name or relative path=path "Report Template") -> (appended path=w97:path)
            n37 = call <vilib>:"Recursive File List.vi"("error in (no error)"=w99, "Folder Path"=w97) -> ("error out"=w98:errorcluster, "All Files in Dir"=w96:path[], "dup Folder Path"=w95:path)  [unwired: 5 in, 2 out]
            n38 = Path To String(path=w95) -> (string=w94:string)
            n39 = Concatenate Strings(w94, "\\" ("string")) -> (w92:string)
            n40 = for {
              tunnel: w96 -> [w110] mode=indexing
              tunnel: w92 -> [w108]
              tunnel: [w107] -> w91 mode=indexing
              n41 = Path To String(path=w110) -> (string=w109:string)
              n42 = Search and Replace String(input string=w109, search string=w108) -> (result string=w107:string)  [unwired: 6 in, 3 out]
            }
            n43 = property on="ListBox.Output Set" class="CmbBox"("Strings[]"=w91) -> ()  [unwired: 2 in, 2 out]
          }
          frame "Get procedure list" {
            n44 = call "FGV - Data Path.vi"("FGV State"=State_-_FGV."Read", "Error In"=w114) -> ("Error Out"=w113:errorcluster, "Path Out"=w112:path)  [unwired: 8 in]
            n45 = Build Path(base path=w112, name or relative path=path "Template Excel") -> (appended path=w121:path)
            n46 = Path To String(path=w121) -> (string=w119:string)
            n47 = call <vilib>:"Recursive File List.vi"("Continue Recursing on Error? (F)"=TRUE, "Folder Path"=w121) -> ("All Files in Dir"=w122:path[])  [unwired: 5 in, 4 out]
            n48 = Concatenate Strings(w119, "\\" ("string")) -> (w117:string)
            n49 = Path To String(path=w122) -> (string=w116:string[])
            n50 = for {
              tunnel: w116 -> [w128] mode=indexing
              tunnel: w117 -> [w127]
              tunnel: [w126] -> w120 mode=indexing
              n51 = Search and Replace String(input string=w128, search string=w127) -> (result string=w126:string)  [unwired: 6 in, 3 out]
            }
            n52 = property on="Procedure No./Ref." class="CmbBox"("Strings[]"=w120) -> ()  [unwired: 2 in, 2 out]
          }
          frame "Idle" {
            n53 = Unbundle By Name(w132) -> ("Event Ref"=w131:refnum<event-registration>)
            n54 = event shown="[11] \"Search\": Value Change" {
              selector: w131 -> [_ _ _ _ _ _ _ _ _ _ _ _ _ _ _ _ _ _ _ _ _ _ _ _ _ _ _ _]
              dyn-events: [_ _ _ _ _ _ _ _ _ _ _ _ _ _ _ _ _ _ _ _ _ _ _ _ _ _ _ _] -> w129
              timeout: _ -> [_ _ _ _ _ _ _ _ _ _ _ _ _ _ _ _ _ _ _ _ _ _ _ _ _ _ _ _]
              tunnel: [w141 w144 w147 w165 w177 w180 w195 w213 w229 w250 w259 w280 w286 w290 w294 w303 w306 w324 w349 w358 w381 w390 w411 w421 w436 w454 w459 w470] -> w138
              tunnel: w137 -> [w141 w144 w153 w171 w177 w180 w195 w213 w229 w250 w259 w280 w286 w290 w295 w303 w312 w328 w355 w365 w383 w392 w418 w428 w437 w454 w460 w471]
              tunnel: [w139 w142 Setup_-_State."Get product info" Setup_-_State."Get Sequence List" Setup_-_State."Get procedure list" Setup_-_State."Get Sequence List" Setup_-_State."Idle" Setup_-_State."Idle" Setup_-_State."Idle" Setup_-_State."Idle" Setup_-_State."Idle" Setup_-_State."Idle" Setup_-_State."Idle" Setup_-_State."Idle" Setup_-_State."Get Transaction Info" Setup_-_State."Idle" Setup_-_State."Idle" Setup_-_State."Idle" Setup_-_State."Idle" Setup_-_State."Idle" Setup_-_State."Idle" Setup_-_State."Idle" Setup_-_State."Idle" Setup_-_State."Idle" Setup_-_State."Idle" Setup_-_State."Close" Setup_-_State."Idle" Setup_-_State."Idle"] -> w135
              tunnel: [w140 w143 w155 w167 w176 w179 w188 w206 w227 w248 w265 w283 w285 w289 w297 w302 w315 w329 w356 w366 w384 w394 w420 w430 w442 w453 w461 w472] -> w134
              tunnel: w132 -> [w140 w143 w157 w174 w176 w179 w189 w207 w228 w249 w267 w283 w285 w289 w297 w302 w315 w329 w356 w366 w384 w394 w420 w430 w442 w453 w461 w472]
              tunnel: w133 -> [w139 w142 _ _ _ _ _ _ _ _ _ _ _ _ _ _ _ _ _ _ _ _ _ _ _ _ _ _]
              event Timeout {
                n55 = event-data() -> ()  [unwired: 1 in, 1 out]
              }
              event "Stop": Value Change {
                n56 = event-data() -> ()  [unwired: 1 in, 6 out]
              }
              event "Product Category": Value Change {
                n57 = event-data() -> ("NewVal"=w150:string, "CtlRef"=w154:refnum<vi>)  [unwired: 1 in]
                n58 = property class="CmbBox"(reference=w154, error in=w153) -> (reference out=w148:refnum<vi>, error out=w149:errorcluster, "Strings[]"=w146:string[])
                n59 = Bundle By Name(cluster=w157, "Product Category"=w150) -> (w155:T11)
                n60 = call "Gen - Remove Empty String Array.vi"("Data Array"=w146) -> ("Data Out"=w145:string[])  [unwired: 10 in]
                n61 = call "Search Unsorted 1D Array.vim"("element"=w150, "unsorted 1D array"=w145) -> ("index of element"=w152:i32)  [unwired: 9 in]
                n62 = Less Than 0?(x=w152) -> (x < 0?=w151:bool)
                n63 = case shown="True" w151 {
                  tunnel: w145 -> [_ w164]
                  tunnel: w150 -> [_ w163]
                  tunnel: w149 -> [w158 w162]
                  tunnel: w148 -> [_ w161]
                  tunnel: [w158 w159] -> w147
                  frame False {
                  }
                  frame True {
                    n64 = Insert Into Array(array=w164, new element=w163) -> (w160:string[])  [unwired: 1 in]
                    n65 = property class="CmbBox"(reference=w161, error in=w162, "Strings[]"=w160) -> (error out=w159:errorcluster)  [unwired: 1 out]
                  }
                }
              }
              event "Procedure No./Ref.": Value Change {
                n66 = event-data() -> ("NewVal"=w166:string, "CtlRef"=w172:refnum<vi>)  [unwired: 1 in]
                n67 = property class="CmbBox"(reference=w172, error in=w171) -> (error out=w165:errorcluster, "Strings[]"=w169:string[])  [unwired: 1 out]
                n68 = call "Gen - Remove Empty String Array.vi"("Data Array"=w169) -> ("Data Out"=w168:string[])  [unwired: 10 in]
                n69 = Bundle By Name(cluster=w174, "Procedure No."=w166) -> (w167:T11)
                n70 = call "Search Unsorted 1D Array.vim"("element"=w166, "unsorted 1D array"=w168) -> ("index of element"=w170:i32)  [unwired: 9 in]
                n71 = Less Than 0?(x=w170) -> ()  [unwired: 1 out]
              }
              event "Procedure No./Ref.": Operate Menu Activation {
                n72 = event-data() -> ()  [unwired: 1 in, 4 out]
              }
              event "Load Excel": Value Change {
                n73 = event-data() -> ()  [unwired: 1 in, 6 out]
              }
              event Value Change {
                n74 = event-data() -> ()  [unwired: 1 in, 6 out]
                n75 = local read "Setup-Sequence Data"() -> (w183:T1)
                n76 = Unbundle By Name(w189) -> ("Bool Tracker.Bool.SelectSeq"=w187:bool)
                n77 = Unbundle By Name(w183) -> ("Array"=w184:T2[])
                n78 = Not(x=w187) -> (.not. x?=w185:bool)
                n79 = Bundle By Name(cluster=w189, "Bool Tracker.Bool.SelectSeq"=w185) -> (w188:T11)
                n80 = for {
                  tunnel: w184 -> [w198] mode=indexing
                  tunnel: w185 -> [w197]
                  tunnel: [w196] -> w182 mode=indexing
                  n81 = Bundle By Name(cluster=w198, "Seq.Select"=w197) -> (w196:T2)
                }
                n82 = Select(t="Unsel." ("Label.SelectSeq"), s=w185, f="Select") -> (s? t:f=w194:string)
                n83 = local read "Setup-Sequence Data"() -> (w191:T1)
                n84 = Bundle By Name(cluster=w191, "Label.SelectSeq"=w194) -> (w190:T1)
                n85 = local write "Setup-Sequence Data"(w190) -> ()
                n86 = Bundle By Name(cluster=w183, "Array"=w182) -> (w181:T1)
                n87 = local write "Setup-Sequence Data"(w181) -> ()
              }
              event Value Change {
                n88 = event-data() -> ()  [unwired: 1 in, 6 out]
                n89 = local read "Setup-Sequence Data"() -> (w202:T1)
                n90 = Unbundle By Name(w207) -> ("Bool Tracker.Bool.RunSeq"=w205:bool)
                n91 = Unbundle By Name(w202) -> ("Array"=w201:T2[])
                n92 = Not(x=w205) -> (.not. x?=w203:bool)
                n93 = for {
                  tunnel: w203 -> [w216]
                  tunnel: [w215] -> w200 mode=indexing
                  tunnel: w201 -> [w214] mode=indexing
                  n94 = Bundle By Name(cluster=w214, "Seq.Run"=w216) -> (w215:T2)
                }
                n95 = Bundle By Name(cluster=w207, "Bool Tracker.Bool.RunSeq"=w203) -> (w206:T11)
                n96 = Select(t="Run" ("Label.SelectSeq"), s=w203, f="Run") -> (s? t:f=w212:string)
                n97 = local read "Setup-Sequence Data"() -> (w209:T1)
                n98 = Bundle By Name(cluster=w209, "Label.RunSeq"=w212) -> (w208:T1)
                n99 = local write "Setup-Sequence Data"(w208) -> ()
                n100 = Bundle By Name(cluster=w202, "Array"=w200) -> (w199:T1)
                n101 = local write "Setup-Sequence Data"(w199) -> ()
              }
              event Value Change {
                n102 = event-data() -> ()  [unwired: 1 in, 6 out]
                n103 = local read "Setup-Sequence Data"() -> (w219:T1)
                n104 = Unbundle By Name(w219) -> ("Array"=w220:T2[])
                n105 = Unbundle By Name(w228) -> ("Bool Tracker.Bool.TestSeq"=w226:bool)
                n106 = for {
                  tunnel: w220 -> [w237] mode=indexing
                  tunnel: [w236] -> w224 mode=indexing
                  n107 = Unbundle By Name(w237) -> ("Seq.TestSequence"=w235:string)
                  n108 = Bundle("Seq.TestSequence"=w235, "Setup - Sequence Data"=w237) -> (w236:T21)  [unwired: 1 in]
                }
                n109 = Not(x=w226) -> (.not. x?=w222:bool)
                n110 = Bundle By Name(cluster=w228, "Bool Tracker.Bool.TestSeq"=w222) -> (w227:T11)
                n111 = call "Sort 1D Array.vim"("unsorted array"=w224) -> ("sorted array"=w223:T22)  [unwired: 10 in]
                n112 = for {
                  tunnel: w223 -> [w234] mode=indexing
                  tunnel: [w233] -> w221 mode=indexing
                  n113 = Unbundle(w234) -> ("Setup - Sequence Data"=w233:T2)  [unwired: 1 out]
                }
                n114 = case shown="False" w222 {
                  tunnel: w221 -> [w230 w232]
                  tunnel: [w230 w231] -> w218
                  frame False {
                  }
                  frame True {
                    n115 = Reverse 1D Array(array=w232) -> (reversed array=w231:T2[])
                  }
                }
                n116 = Bundle By Name(cluster=w219, "Array"=w218) -> (w217:T1)
                n117 = local write "Setup-Sequence Data"(w217) -> ()
              }
              event Value Change {
                n118 = event-data() -> ()  [unwired: 1 in, 6 out]
                n119 = local read "Setup-Sequence Data"() -> (w240:T1)
                n120 = Unbundle By Name(w249) -> ("Bool Tracker.Bool.NoSeq"=w247:bool)
                n121 = Unbundle By Name(w240) -> ("Array"=w241:T2[])
                n122 = Not(x=w247) -> (.not. x?=w243:bool)
                n123 = for {
                  tunnel: w241 -> [w257] mode=indexing
                  tunnel: [w256] -> w245 mode=indexing
                  n124 = Unbundle By Name(w257) -> ("Seq.No"=w258:string)
                  n125 = Bundle("Seq.No"=w258, "Setup - Sequence Data"=w257) -> (w256:T23)  [unwired: 1 in]
                }
                n126 = Bundle By Name(cluster=w249, "Bool Tracker.Bool.NoSeq"=w243) -> (w248:T11)
                n127 = call "Sort 1D Array.vim"("unsorted array"=w245) -> ("sorted array"=w244:T24)  [unwired: 10 in]
                n128 = for {
                  tunnel: w244 -> [w255] mode=indexing
                  tunnel: [w254] -> w242 mode=indexing
                  n129 = Unbundle(w255) -> ("Setup - Sequence Data"=w254:T2)  [unwired: 1 out]
                }
                n130 = case shown="True" w243 {
                  tunnel: w242 -> [w251 w253]
                  tunnel: [w251 w252] -> w239
                  frame False {
                  }
                  frame True {
                    n131 = Reverse 1D Array(array=w253) -> (reversed array=w252:T2[])
                  }
                }
                n132 = Bundle By Name(cluster=w240, "Array"=w239) -> (w238:T1)
                n133 = local write "Setup-Sequence Data"(w238) -> ()
              }
              event "ComboBox.SelectTestSequence": Value Change {
                n134 = event-data() -> ("NewVal"=w261:string)  [unwired: 1 in]
                n135 = Unbundle By Name(w267) -> ("Seq.AllList"=w266:T16)
                n136 = To Lower Case(string=w261) -> (all lower case string=w260:string)
                n137 = case shown="\"all\"" w260 {
                  tunnel: w266 -> [w271 w278]
                  tunnel: w261 -> [w270 _]
                  tunnel: [w269 T16 []] -> w264
                  tunnel: [w268 w278] -> w263
                  frame Default {
                    n138 = for {
                      tunnel: w271 -> [w274] mode=indexing
                      tunnel: w270 -> [w275]
                      tunnel: [w274] -> w268 mode=indexing if=w272
                      tunnel: [w274] -> w269 mode=indexing if=w273
                      n139 = Unbundle By Name(w274) -> ("Seq.TestSequence"=w276:string)
                      n140 = Equal?(x=w276, y=w275) -> (x = y?=w272:bool)
                      n141 = Not(x=w272) -> (.not. x?=w273:bool)
                    }
                  }
                  frame "all" {
                  }
                }
                n142 = Bundle By Name(cluster=w267, "Seq.ShownList"=w263, "Seq.HiddenList"=w264) -> (w265:T11)
              }
              event "Search": Value Change {
                w279 = T17."Disabled and Grayed Out" ("Disabled")
                n143 = event-data() -> ()  [unwired: 1 in, 6 out]
                n144 = call "DB UI - Search-Load Setup.vi"("error in (no error)"=w280) -> ("1D Results"=→"1D Results":string[])  [unwired: 7 in, 3 out]
                n145 = property on="Order Number" class="Str"("DisabledEnum"=w279) -> ()  [unwired: 2 in, 2 out]
                n146 = property on="Ref Order No." class="Str"("DisabledEnum"=w279) -> ()  [unwired: 2 in, 2 out]
                n147 = property on="Customer Description" class="Str"("DisabledEnum"=w279) -> ()  [unwired: 2 in, 2 out]
                n148 = property on="Project" class="Str"("DisabledEnum"=w279) -> ()  [unwired: 2 in, 2 out]
                n149 = property on="Material" class="Str"("DisabledEnum"=w279) -> ()  [unwired: 2 in, 2 out]
                n150 = property on="Procedure No./Ref." class="CmbBox"("DisabledEnum"=w279) -> ()  [unwired: 2 in, 2 out]
                n151 = property on="Material Description" class="Str"("DisabledEnum"=w279) -> ()  [unwired: 2 in, 2 out]
              }
              event "Copy Transaction": Value Change {
                n152 = event-data() -> ()  [unwired: 1 in, 6 out]
              }
              event "NewTransaction": Value Change {
                w287 = T17."Enabled" ("Disabled")
                n153 = event-data() -> ()  [unwired: 1 in, 6 out]
                n154 = property on="Order Number" class="Str"("DisabledEnum"=w287) -> ()  [unwired: 2 in, 2 out]
                n155 = property on="Ref Order No." class="Str"("DisabledEnum"=w287) -> ()  [unwired: 2 in, 2 out]
                n156 = property on="Customer Description" class="Str"("DisabledEnum"=w287) -> ()  [unwired: 2 in, 2 out]
                n157 = property on="Project" class="Str"("DisabledEnum"=w287) -> ()  [unwired: 2 in, 2 out]
                n158 = property on="Material" class="Str"("DisabledEnum"=w287) -> ()  [unwired: 2 in, 2 out]
                n159 = property on="Procedure No./Ref." class="CmbBox"("DisabledEnum"=w287) -> ()  [unwired: 2 in, 2 out]
                n160 = property on="Material Description" class="Str"("DisabledEnum"=w287) -> ()  [unwired: 2 in, 2 out]
              }
              event "Save Transaction": Value Change {
                n161 = event-data() -> ()  [unwired: 1 in, 6 out]
                n162 = Unbundle By Name(w297) -> ("Seq.AllList"=w296:T16)
                n163 = for {
                  tunnel: w296 -> [w300] mode=indexing
                  tunnel: w296 -> [w299] mode=indexing
                  tunnel: [w299] -> w293 mode=indexing if=w298
                  n164 = Unbundle By Name(w300) -> ("Seq.Run"=w298:bool)
                }
                n165 = call "eFGV - Sequence Data.vi"("States"=State_-_eFGV."Write", "Error In"=w295, "Sequence Data"=w293) -> ("Error Out"=w294:errorcluster)  [unwired: 6 in, 2 out]
              }
              event "Edit Transaction": Value Change {
                n166 = event-data() -> ()  [unwired: 1 in, 6 out]
              }
              event "Test System": Value Change {
                n167 = event-data() -> ("NewVal"=w309:string, "CtlRef"=w313:refnum<vi>)  [unwired: 1 in]
                n168 = property class="CmbBox"(reference=w313, error in=w312) -> (reference out=w307:refnum<vi>, error out=w308:errorcluster, "Strings[]"=w305:string[])
                n169 = call "Gen - Remove Empty String Array.vi"("Data Array"=w305) -> ("Data Out"=w304:string[])  [unwired: 10 in]
                n170 = call "Search Unsorted 1D Array.vim"("element"=w309, "unsorted 1D array"=w304) -> ("index of element"=w311:i32)  [unwired: 9 in]
                n171 = Less Than 0?(x=w311) -> (x < 0?=w310:bool)
                n172 = case shown="True" w310 {
                  tunnel: w304 -> [_ w322]
                  tunnel: w309 -> [_ w321]
                  tunnel: w308 -> [w316 w320]
                  tunnel: w307 -> [_ w319]
                  tunnel: [w316 w317] -> w306
                  frame False {
                  }
                  frame True {
                    n173 = Insert Into Array(array=w322, new element=w321) -> (w318:string[])  [unwired: 1 in]
                    n174 = property class="CmbBox"(reference=w319, error in=w320, "Strings[]"=w318) -> (error out=w317:errorcluster)  [unwired: 1 out]
                  }
                }
              }
              event "Add SN": Value Change {
                n175 = event-data() -> ()  [unwired: 1 in, 6 out]
                n176 = property on="Input SN" class="Str"(error in=w328) -> (error out=w327:errorcluster, "Value"=w325:string)  [unwired: 1 in, 1 out]
                n177 = Empty String/Path?(string/path=w325) -> (empty?=w326:bool)
                n178 = case shown="False" w326 {
                  tunnel: w327 -> [w332 w346]
                  tunnel: w325 -> [w334 _]
                  tunnel: [w333 w346] -> w324
                  frame False {
                    n179 = property on="List SN" class="LstBox (strict)"(error in=w332) -> (error out=w331:errorcluster, "Item Names"=w330:string[])  [unwired: 1 in, 1 out]
                    n180 = call "Search Unsorted 1D Array.vim"("element"=w334, "unsorted 1D array"=w330) -> ("index of element"=w336:i32)  [unwired: 9 in]
                    n181 = Less Than 0?(x=w336) -> (x < 0?=w335:bool)
                    n182 = case shown="True" w335 {
                      tunnel: w331 -> [w337 w341]
                      tunnel: w330 -> [_ w345]
                      tunnel: w334 -> [_ w344]
                      tunnel: [w337 w342] -> w333
                      frame False {
                        n183 = One Button Dialog(message="Serial Number already exist") -> ()  [unwired: 1 in, 1 out]
                      }
                      frame True {
                        n184 = Insert Into Array(array=w345, new element=w344) -> (w339:string[])  [unwired: 1 in]
                        n185 = property on="List SN" class="LstBox (strict)"(error in=w341, "Item Names"=w339) -> (error out=w340:errorcluster)  [unwired: 1 in, 1 out]
                        n186 = property on="Input SN" class="Str"(error in=w340, "Value"="" ("Input SN")) -> (error out=w342:errorcluster)  [unwired: 1 in, 1 out]
                      }
                    }
                  }
                  frame True {
                    n187 = One Button Dialog(message="Serial number empty") -> ()  [unwired: 1 in, 1 out]
                  }
                }
              }
              event "List SN": Mouse Down {
                n188 = event-data() -> ("CtlRef"=w354:refnum<vi>)  [unwired: 1 in, 7 out]
                n189 = property class="LstBox (strict)"(reference=w354, error in=w355) -> (error out=w351:errorcluster, "FocusRow"=w352:i32, "Item Names"=w353:string[])  [unwired: 1 out]
                n190 = Index Array(array=w353, index=w352) -> (element=w350:string)
                n191 = property on="Input SN" class="Str"(error in=w351, "Value"=w350) -> (error out=w349:errorcluster)  [unwired: 1 in, 1 out]
              }
              event "Remove SN": Value Change {
                n192 = event-data() -> ()  [unwired: 1 in, 6 out]
                n193 = property on="List SN" class="LstBox (strict)"(error in=w365) -> (error out=w364:errorcluster, "Item Names"=w360:string[])  [unwired: 1 in, 1 out]
                n194 = property on="Input SN" class="Str"(error in=w364) -> (error out=w361:errorcluster, "Value"=w363:string)  [unwired: 1 in, 1 out]
                n195 = call "Search Unsorted 1D Array.vim"("element"=w363, "unsorted 1D array"=w360) -> ("index of element"=w359:i32)  [unwired: 9 in]
                n196 = Less Than 0?(x=w359) -> (x < 0?=w362:bool)
                n197 = case shown="False" w362 {
                  tunnel: w361 -> [w370 w375]
                  tunnel: w360 -> [w374 _]
                  tunnel: w359 -> [w373 _]
                  tunnel: [w367 w375] -> w358
                  frame False {
                    n198 = Delete From Array(array=w374, length=1, index=w373) -> (array with subset deleted=w371:string[])  [unwired: 1 out]
                    n199 = property on="List SN" class="LstBox (strict)"(error in=w370, "Item Names"=w371) -> (error out=w369:errorcluster)  [unwired: 1 in, 1 out]
                    n200 = property on="Input SN" class="Str"(error in=w369, "Value"="" ("Input SN")) -> (error out=w367:errorcluster)  [unwired: 1 in, 1 out]
                  }
                  frame True {
                    n201 = One Button Dialog(message="No matching SN to remove") -> ()  [unwired: 1 in, 1 out]
                  }
                }
              }
              event "Rework": Value Change {
                n202 = event-data() -> ("NewVal"=w380:bool)  [unwired: 1 in]
                n203 = case shown="False" w380 {
                  tunnel: [FALSE ("Visible") TRUE ("Visible")] -> w379
                  tunnel: [T17."Disabled" ("Disabled") T17."Enabled" ("Disabled")] -> w378
                  frame False {
                  }
                  frame True {
                  }
                }
                n204 = property on="NCR No." class="Str"(error in=w383, "Visible"=w379, "DisabledEnum"=w378) -> (error out=w382:errorcluster)  [unwired: 1 in, 1 out]
                n205 = property on="Ref Order No." class="Str"(error in=w382, "Visible"=w379, "DisabledEnum"=w378) -> (error out=w381:errorcluster)  [unwired: 1 in, 1 out]
              }
              event "Add Sensor": Value Change {
                n206 = event-data() -> ()  [unwired: 1 in, 5 out]
                n207 = call "Popup - Add Sensor.vi"() -> ("Output Sensor"=w389:T25, "Cancelled?"=w391:bool)  [unwired: 10 in]
                n208 = case shown="False" w391 {
                  tunnel: w392 -> [w409 w410]
                  tunnel: [w405 w410] -> w390
                  tunnel: w389 -> [w404 _]
                  frame False {
                    n209 = Unbundle By Name(w404) -> ("Type"=w396:string, "ID"=w397:string, "Description"=w398:string, "Serial No."=w399:string, "Low Pressure?"=w403:bool)
                    n210 = Select(t="Y", s=w403, f="N") -> (s? t:f=w400:string)
                    n211 = Build Array(w396, w397, w398, w399, w400) -> (w395:string[])
                    n212 = property on="Table.Sensor" class="MCListbox (strict)"(error in=w409) -> (error out=w407:errorcluster, "ItemNames"=w408:string[][])  [unwired: 1 in, 1 out]
                    n213 = Insert Into Array(array=w408, new element=w395) -> (w406:string[][])  [unwired: 2 in]
                    n214 = property on="Table.Sensor" class="MCListbox (strict)"(error in=w407, "ItemNames"=w406) -> (error out=w405:errorcluster)  [unwired: 1 in, 1 out]
                  }
                  frame True {
                  }
                }
              }
              event "Remove Sensor": Value Change {
                n215 = event-data() -> ()  [unwired: 1 in, 5 out]
                n216 = property on="Table.Sensor" class="MCListbox (strict)"(error in=w418) -> (error out=w417:errorcluster, "FocusRow"=w414:i32)  [unwired: 1 in, 1 out]
                n217 = property on="Table.Sensor" class="MCListbox (strict)"(error in=w417) -> (error out=w412:errorcluster, "ItemNames"=w416:string[][])  [unwired: 1 in, 1 out]
                n218 = Delete From Array(array=w416, length=1, index (row)=w414) -> (array with subset deleted=w413:string[][])  [unwired: 1 in, 1 out]
                n219 = property on="Table.Sensor" class="MCListbox (strict)"(error in=w412, "ItemNames"=w413) -> (error out=w411:errorcluster)  [unwired: 1 in, 1 out]
              }
              event "Remove Additional Ref Procedure": Value Change {
                n220 = event-data() -> ()  [unwired: 1 in, 5 out]
                n221 = property on="Table.Procedure No./Ref." class="MCListbox (strict)"(error in=w428) -> (error out=w427:errorcluster, "FocusRow"=w424:i32)  [unwired: 1 in, 1 out]
                n222 = property on="Table.Procedure No./Ref." class="MCListbox (strict)"(error in=w427) -> (error out=w422:errorcluster, "ItemNames"=w426:string[][])  [unwired: 1 in, 1 out]
                n223 = Delete From Array(array=w426, length=1, index (row)=w424) -> (array with subset deleted=w423:string[][])  [unwired: 1 in, 1 out]
                n224 = property on="Table.Procedure No./Ref." class="MCListbox (strict)"(error in=w422, "ItemNames"=w423) -> (error out=w421:errorcluster)  [unwired: 1 in, 1 out]
              }
              event "Add Additional Ref Procedure": Value Change {
                n225 = event-data() -> ()  [unwired: 1 in, 5 out]
                n226 = local read "Listbox.Additional Procedures No./Ref."() -> (w434:string)
                n227 = local read "Listbox.Rev."() -> (w433:string)
                n228 = local read "Listbox.PSL"() -> (w435:string)
                n229 = Empty String/Path?(string/path=w434) -> (empty?=w441:bool)
                n230 = Empty String/Path?(string/path=w433) -> (empty?=w440:bool)
                n231 = Empty String/Path?(string/path=w435) -> (empty?=w439:bool)
                n232 = Build Array(w434, w433, w435) -> (w432:string[])
                n233 = Compound Arithmetic op=OR(w441, w440, w439) -> (w431:bool)
                n234 = case shown="False" w431 {
                  tunnel: w437 -> [w449 w451]
                  tunnel: [w444 w451] -> w436
                  tunnel: w432 -> [w447 _]
                  frame False {
                    w443 = "" ("Listbox.Additional Procedures No./Ref.")
                    n235 = property on="Table.Procedure No./Ref." class="MCListbox (strict)"(error in=w449) -> (error out=w445:errorcluster, "ItemNames"=w448:string[][])  [unwired: 1 in, 1 out]
                    n236 = local write "Listbox.Additional Procedures No./Ref."(w443) -> ()
                    n237 = Insert Into Array(array=w448, new element=w447) -> (w446:string[][])  [unwired: 2 in]
                    n238 = property on="Table.Procedure No./Ref." class="MCListbox (strict)"(error in=w445, "ItemNames"=w446) -> (error out=w444:errorcluster)  [unwired: 1 in, 1 out]
                    n239 = local write "Listbox.Rev."(w443) -> ()
                    n240 = local write "Listbox.PSL"(w443) -> ()
                  }
                  frame True {
                    n241 = One Button Dialog(message="EMPTY PARAMETER") -> ()  [unwired: 1 in, 1 out]
                  }
                }
              }
              event User Event {
                n242 = event-data() -> ()  [unwired: 1 in, 5 out]
              }
              event "Enum.Max Start Hold Pressure": Value Change {
                n243 = event-data() -> ("NewVal"=w458:enum16{"%", "psi"})  [unwired: 1 in]
                n244 = case shown="\"%\", Default" w458 {
                  tunnel: [100.0 ("Data Entry Limits:Maximum") 30000.0 ("Data Entry Limits:Maximum")] -> w457
                  tunnel: [0.0 ("Data Entry Limits:Minimum") 0.0 ("Data Entry Limits:Minimum")] -> w456
                  frame "%", Default {
                  }
                  frame "psi" {
                  }
                }
                n245 = property on="Max Start Hold Pressure" class="DigNum (strict)"(error in=w460, "Maximum"=w457, "Minimum"=w456) -> (error out=w459:errorcluster)  [unwired: 1 in, 1 out]
              }
              event "Enum.Permitted Hold Pressure Drop": Value Change {
                n246 = event-data() -> ("NewVal"=w469:enum16{"%", "psi"})  [unwired: 1 in]
                n247 = case shown="\"%\", Default" w469 {
                  tunnel: [100.0 ("Data Entry Limits:Maximum") 30000.0 ("Data Entry Limits:Maximum")] -> w468
                  tunnel: [0.0 ("Data Entry Limits:Minimum") 0.0 ("Data Entry Limits:Minimum")] -> w467
                  frame "%", Default {
                  }
                  frame "psi" {
                  }
                }
                n248 = property on="Permitted Hold Pressure Drop" class="DigNum (strict)"(error in=w471, "Maximum"=w468, "Minimum"=w467) -> (error out=w470:errorcluster)  [unwired: 1 in, 1 out]
              }
            }
            n249 = Bundle By Name(cluster=w134, "Event Ref"=w129) -> (w130:T11)
          }
          frame "Get product info" {
            n250 = call "FGV - Data Path.vi"("FGV State"=State_-_FGV."Read", "Error In"=w482) -> ("Error Out"=w484:errorcluster, "Path Out"=w485:path)  [unwired: 8 in]
            n251 = Unbundle By Name(w480) -> ("Product Category"=w479:string)
            n252 = Build Path(base path=w485, name or relative path="Data\\Procedure") -> (appended path=w488:path)
            n253 = Build Path(base path=w488, name or relative path="Product Category.ini") -> (appended path=w486:path)
            n254 = call <vilib>:"Open Config Data.vi"("error in (no error)"=w484, "configuration file path"=w486) -> ("error out"=w501:errorcluster, "refnum"=w500:T20)  [unwired: 7 in, 1 out]
            n255 = for {
              tunnel: w501 -> [w508]
              tunnel: w500 -> [w507]
              tunnel: w479 -> [w506]
              tunnel: string[] ["Procedure No", "Rev", "PSL", "Working Pressure"] -> [w505] mode=indexing
              tunnel: [w504] -> w494 mode=indexing
              tunnel: [w503] -> w498
              tunnel: [w502] -> w497
              n256 = call-poly <vilib>:"Read Key.vi"("section"=w506, "error in (no error)"=w508, "key"=w505, "refnum"=w507) -> ("error out"=w503:errorcluster, "value"=w504:string, "refnum out"=w502:T20)  [unwired: 4 in, 1 out]
            }
            n257 = Index Array(array=w494) -> (element #2=w493:string, element #3=w492:string, element #4=w491:string)  [unwired: 4 in, 1 out]
            n258 = call <vilib>:"Close Config Data.vi"("error in (no error)"=w498, "refnum"=w497) -> ("error out"=w483:errorcluster)  [unwired: 8 in, 1 out]
            n259 = property on="Rev." class="Str"(error in=w483, "Value"=w493) -> (error out=w496:errorcluster)  [unwired: 1 in, 1 out]
            n260 = property on="PSL" class="Str"(error in=w496, "Value"=w492) -> (error out=w495:errorcluster)  [unwired: 1 in, 1 out]
            n261 = property on="Working Pressure" class="Str"(error in=w495, "Value"=w491) -> (error out=w481:errorcluster)  [unwired: 1 in, 1 out]
          }
          frame "Read sequence csv" {
            n262 = disable-structure shown="Enabled" {
              disable-tunnel: [w520 w527] -> w510
              disable-tunnel: w509 -> [w519 w527]
              frame Disabled {
                (unwired) path "C:/Users/SNG_THINKPAD/Documents/g159-one-subsea-test-pressure-monitoring-system/VI/HMI/Data/Data/Procedure" ("configuration file path")
                n263 = call "FGV - Data Path.vi"("FGV State"=State_-_FGV."Read", "Error In"=w519) -> ("Error Out"=w514:errorcluster, "Path Out"=w517:path)  [unwired: 8 in]
                n264 = Build Path(base path=w517, name or relative path="Data\\Procedure") -> (appended path=w515:path)
                n265 = Concatenate Strings(".csv" ("string")) -> (w525:string)  [unwired: 1 in]
                n266 = Build Path(base path=w515, name or relative path=w525) -> (appended path=w526:path)
                n267 = call-poly <vilib>:"Read Delimited Spreadsheet.vi"("file path (dialog if empty)"=w526, "error in (no error)"=w514) -> ("all rows"=w523:string[][], "error out"=w521:errorcluster)  [unwired: 8 in, 4 out]
                n268 = call "Get sequence list.vi"("all rows"=w523) -> ("Output sequence"=w522:T16)
              }
              frame Enabled {
              }
            }
          }
          frame "Get Sequence List" {
            n269 = property on="Procedure No./Ref." class="CmbBox"() -> ("Value"=w531:string)  [unwired: 2 in, 2 out]
            n270 = Unbundle By Name(w533) -> ("File String"=w532:string[])
            n271 = for {
              tunnel: w532 -> [w540] mode=indexing
              tunnel: w531 -> [w541]
              tunnel: [w540] -> w530
              tunnel: [w538] -> w528
              stop <- w538 continue-if-true
              n272 = Match Pattern(string=w540, regular expression=w541) -> (match substring=w539:string)  [unwired: 1 in, 3 out]
              n273 = Empty String/Path?(string/path=w539) -> (empty?=w538:bool)
            }
            n274 = String To Path(string=w530) -> (path=w529:path)
            n275 = case shown="False" w528 {
              tunnel: w537 -> [w561 w563]
              tunnel: [w545 w563] -> w536
              tunnel: w529 -> [w546 _]
              tunnel: w533 -> [w548 w562]
              tunnel: [w548 w562] -> w535
              frame False {
                n276 = local read "Setup-Sequence Data"() -> (w544:T1)
                n277 = call <vilib>:"Create Report.vi"("window state (normal)"=T18."no change", "report type"=Report_Type."Excel", "template (empty)"=w546, "error in (no error)"=w561) -> ("report out"=w557:refnum<class "NI_report.lvclass">, "error out"=w558:errorcluster)  [unwired: 10 in]
                n278 = call <vilib>:"Excel Get Worksheet.vi"("report in"=w557, "worksheet index (0)"=0, "error in (no error)"=w558) -> ("report out"=w554:refnum<class "NI_report.lvclass">, "error out"=w555:errorcluster)  [unwired: 11 in]
                n279 = call-poly <vilib>:"Excel Get Data.vi"("report in"=w554, "data type"=string[][] [], "error in (no error)"=w555) -> ("report out"=w551:refnum<class "NI_report.lvclass">, "data"=w547:string[][], "error out"=w552:errorcluster)  [unwired: 10 in]
                n280 = call "Sequence Data 2d Array to Cluster.vi"("data"=w547) -> ("Array"=w543:T2[])  [unwired: 4 in, 5 out]
                n281 = Bundle By Name(cluster=w544, "Array"=w543) -> (w542:T1)
                n282 = call-dynamic "Dispose Report.vi"("report in"=w551, "error in (no error)"=w552) -> ("error out"=w550:errorcluster)  [unwired: 13 in]
                n283 = call "Gen - Get Unique Value.vi"("data"=w547) -> ("Unique Values"=w549:string[])
                n284 = property on="ComboBox.SelectTestSequence" class="CmbBox"(error in=w550, "Strings[]"=w549) -> (error out=w545:errorcluster)  [unwired: 1 in, 1 out]
                n285 = local write "Setup-Sequence Data"(w542) -> ()
              }
              frame True {
              }
            }
          }
          frame "Get Transaction Info" {
            # "#CHECK FOR Data type mismatch"
            n286 = local read "Customer Description"() -> (w569:string)
            n287 = local read "Transaction Number"() -> (w565:string)
            n288 = local read "Material Description"() -> (w573:string)
            n289 = local read "Order Number"() -> (w566:string)
            n290 = local read "Ref Order No."() -> (w576:string)
            n291 = local read "Sales Order"() -> (w571:string)
            n292 = local read "Customer"() -> (w568:string)
            n293 = local read "BOM Rev."() -> (w578:string)
            n294 = local read "Quantity"() -> (w567:u16)
            n295 = local read "NCR No."() -> (w575:string)
            n296 = local read "Item No."() -> (w577:string)
            n297 = local read "Material"() -> (w572:string)
            n298 = local read "Rework"() -> (w574:bool)
            n299 = local read "Project"() -> (w570:string)
            n300 = Bundle("Transaction Number"=w565, "Order Number"=w566, "Quantity"=w567, "Customer"=w568, "Customer Description"=w569, "Project"=w570, "Sales Order"=w571, "Material"=w572, "Material Description"=w573, "Rework"=w574, "NCR No."=w575, "Ref Order No."=w576, "Item No."=w577, "BOM Rev."=w578) -> (w564:T26)  [unwired: 1 in]
            n301 = disable-structure shown="Enabled" {
              disable-tunnel: w581 -> [w586 w587]
              disable-tunnel: [w585 w587] -> w579
              disable-tunnel: w564 -> [w584 _]
              frame Enabled {
                n302 = Bundle By Name(cluster=w586, "Data to Execute.Transaction Info"=w584) -> (w585:T11)
              }
              frame Disabled {
              }
            }
          }
          frame "Get product Info" {
            n303 = local read "Test System Description"() -> (w594:string)
            n304 = local read "Procedure No./Ref."() -> (w592:string)
            n305 = local read "Product Category"() -> (w591:string)
            n306 = local read "Working Pressure"() -> (w595:string)
            n307 = local read "Pressure Unit"() -> (w596:string)
            n308 = local read "Test System"() -> (w593:string)
            n309 = local read "Rev."() -> (w597:string)
            n310 = local read "PSL"() -> (w598:string)
            n311 = Bundle("Product Category"=w591, "Procedure No./Ref."=w592, "Test System"=w593, "Test System Description"=w594, "Working Pressure"=w595, "Pressure Unit"=w596, "Rev."=w597, "PSL"=w598) -> (w589:T27)  [unwired: 1 in]
            n312 = Bundle By Name(cluster=w599, "Data to Execute.Product Info"=w589) -> (w590:T11)
          }
          frame "Get Misc - Additional Refs" {
            n313 = property on="Table.Procedure No./Ref." class="MCListbox (strict)"(error in=w605) -> (error out=w604:errorcluster, "ItemNames"=w602:string[][])  [unwired: 1 in, 1 out]
            n314 = Bundle By Name(cluster=w606, "Data to Execute.Misc - Additional Refs"=w602) -> (w603:T11)
          }
          frame "Get Misc - Sensors" {
            n315 = property on="Table.Sensor" class="MCListbox (strict)"(error in=w611) -> (error out=w610:errorcluster, "ItemNames"=w608:string[][])  [unwired: 1 in, 1 out]
            n316 = Bundle By Name(cluster=w612, "Data to Execute.Misc - Sensors"=w608) -> (w609:T11)
          }
          frame "Get Misc - Tools" {
          }
          frame "Get Misc - Accept Criteria" {
            n317 = local read "Enum.Permitted Hold Pressure Drop"() -> (w624:enum16{"%", "psi"})
            n318 = local read "Enum.Pressure stabilize wait time"() -> (w617:enum16{"seconds", "minutes"})
            n319 = local read "Enum.Max Start Hold Pressure"() -> (w623:enum16{"%", "psi"})
            n320 = local read "Permitted Hold Pressure Drop"() -> (w619:dbl)
            n321 = local read "Pressure stabilize wait time"() -> (w618:dbl)
            n322 = local read "Max Start Hold Pressure"() -> (w622:dbl)
            n323 = Bundle("Max Start Hold Pressure"=w622, "Enum.Max Start Hold Pressure"=w623, "Permitted Hold Pressure Drop"=w619, "Enum.Permitted Hold Pressure Drop"=w624, "Pressure stabilize wait time"=w618, "Enum.Pressure stabilize wait time"=w617) -> (w616:T28)  [unwired: 1 in]
            n324 = Bundle By Name(cluster=w625, "Data to Execute.Acceptance Criteria Info"=w616) -> (w621:T11)
          }
          frame "Get Misc - Execution" {
            n325 = local read "Auto Set Marker"() -> (w631:bool)
            n326 = local read "Auto Stop Test"() -> (w630:bool)
            n327 = Bundle("Auto Set Marker"=w631, "Auto Stop Test"=w630) -> (w628:T29)  [unwired: 1 in]
            n328 = Bundle By Name(cluster=w632, "Data to Execute.Execution Info"=w628) -> (w629:T11)
          }
          frame "Get Misc - Results" {
            n329 = local read "Output Set Description"() -> (w637:string)
            n330 = local read "ListBox.Output Set"() -> (w638:string)
            n331 = Bundle("ListBox.Output Set"=w638, "Output Set Description"=w637) -> (w635:T30)  [unwired: 1 in]
            n332 = Bundle By Name(cluster=w639, "Data to Execute.Results Info"=w635) -> (w636:T11)
          }
          frame "Get Misc - Notes" {
            n333 = local read "Notes"() -> (w642:string)
            n334 = Bundle By Name(cluster=w644, "Data to Execute.Notes"=w642) -> (w643:T11)
          }
          frame "Check Folder Exist" {
            n335 = call "FGV - Data Path.vi"("FGV State"=State_-_FGV."Read", "Error In"=w659) -> ("Error Out"=w655:errorcluster, "Path Out"=w658:path)  [unwired: 8 in]
            n336 = Unbundle By Name(w656) -> ()  [unwired: 1 out]
            n337 = Build Path(base path=w658, name or relative path=path "Results") -> (appended path=w654:path)
            n338 = Build Path(base path=w654, name or relative path="0") -> (appended path=w653:path)
            n339 = call <vilib>:"Check if File or Folder Exists.vi"("error in (no error)"=w655, "path"=w653) -> ("error out"=w652:errorcluster, "file or folder exists?"=w651:bool, "dup path"=w648:path)  [unwired: 7 in]
            n340 = case shown="False" w651 {
              tunnel: w652 -> [w662 w665]
              tunnel: [Setup_-_State."Send to Execute" Setup_-_State."Idle"] -> w650
              tunnel: [w660 w664] -> w649
              tunnel: w648 -> [w661 _]
              frame False {
                n341 = Create Folder(path (use dialog)=w661, error in=w662) -> (error out=w660:errorcluster)  [unwired: 1 in, 2 out]
              }
              frame True {
                n342 = call "Gen - Popup Single Button (Auto Close).vi"("Error in"=w665, "Message in"="Transaction number is already used", "Header"="FILE EXISTS") -> ("Error out"=w664:errorcluster)  [unwired: 7 in, 1 out]
              }
            }
          }
          frame "Send to Execute" {
            n343 = Unbundle By Name(w671) -> ("Data to Execute"=w670:T5)
            n344 = call "eFGV - Data to Execute.vi"("Action"=State_-_eFGV."Write", "Error In"=w674, "Data to Execute"=w670) -> ("Error Out"=w673:errorcluster)  [unwired: 7 in, 1 out]
          }
          frame "Close" {
            n345 = Unbundle By Name(w676) -> ("Event Ref"=w675:refnum<event-registration>)
            n346 = Unregister For Events(event registration refnum=w675, error in=w680) -> (error out=w679:errorcluster)
          }
        }
      }
      frame Error {
        n347 = call <vilib>:"Clear Errors.vi"("error in (no error)"=w684) -> ("error out"=w687:errorcluster)  [unwired: 5 in, 1 out]
        n348 = call "Gen - Get Application Kind.vi"("Error In"=w687) -> ("Error Out"=w683:errorcluster, "Application:Kind"=w686:T31)  [unwired: 9 in]
        n349 = Format Into String(error in=w683, w681) -> (resulting string=w682:string)  [unwired: 2 in, 1 out]
        n350 = case shown="\"Development System\"" w686 {
          tunnel: [w691 w696 w700] -> w685
          tunnel: w684 -> [w691 w693 w698]
          tunnel: w682 -> [_ w692 _]
          frame "invalid app kind", Default {
          }
          frame "Run Time System" {
            n351 = control-ref of="This VI"() -> (w694:refnum<vi>)
            n352 = call "eFGV - Generated Error.vi"("eFGV States"=State_-_eFGV."Write", "Error In"=w693, "State"=w692, "This VI"=w694) -> ("Error Out"=w696:errorcluster)  [unwired: 6 in, 1 out]
          }
          frame "Development System" {
            n353 = call <vilib>:"Simple Error Handler.vi"("error in (no error)"=w698) -> ("error?"=w697:bool, "error out"=w699:errorcluster)  [unwired: 4 in, 3 out]
            n354 = case shown="False" w697 {
              tunnel: [w701 w703] -> w700
              tunnel: w699 -> [w701 w702]
              frame False {
              }
              frame True {
                n355 = call <vilib>:"Clear Errors.vi"("error in (no error)"=w702) -> ("error out"=w703:errorcluster)  [unwired: 5 in, 1 out]
              }
            }
          }
        }
      }
    }
    n356 = Wait (ms)(milliseconds to wait=u32 1) -> ()  [unwired: 1 out]
  }
  n357 = while {
    stop <- FALSE stop-if-true
    # "#HIDDEN"
  }
